vi "20191023_KEK_HEX5_simple.vi"() -> ()   [LabVIEW 2017]
uses:
  <vilib>/DAQmx/create/channels.llb/DAQmx Create Channel (AI-Voltage-Basic).vi
  <vilib>/DAQmx/create/channels.llb/DAQmx Create Channel (AO-Voltage-Basic).vi
  <vilib>/DAQmx/miscellaneous.llb/DAQmx Fill In Error Info.vi
  Lake Shore Cryotronics 218.lvlib
panel:
  out "ref RAW":refnum<file>
  out "ref LSI-D":refnum<file>
  out "ref DAQ":refnum<file>
  in  "CSV filename suffix":string="transfer"
  in  "base path":path=path "C:/Users/TUCAN_rcnp/Desktop/Labview/KEK_20191023_HEX5/EXP"
  out "ref LSI-U":refnum<file>
  out "Cycle #":i32=4
  out "current time":timestamp=timestamp(3655347463.253907 s since 1904-01-01)
  in  "stop":bool
  in  "Tab Control":T1(tab)=enum."config"
  out "error out \n(LSIU)":errorcluster
  out "error out\n(file creation)":errorcluster
  out "error out\n(DAQ config)":errorcluster
  out "error out\n(DAQ OUT)":errorcluster
  out "error out \n(DAQ IN)":errorcluster
  out "error out \n(record LSIU)":errorcluster
  out "error out \n(record DAQ)":errorcluster
  out "error out DAQ close":errorcluster
  out "error out \n(LSID)":errorcluster
  out "error out \n(record LSID)":errorcluster
  out "errors plot cosmetic 1":errorcluster[](array[cluster])
  out "error plot content":errorcluster
  out "error plot cosmetic 2":errorcluster
  in  "comments DAQ (not recorded)":string[](array[string])=["", "", "pressure diff., range : 0-20kPa", "pressure diff., rrange : 0-1kPa", "", "", "The range of this is 0-10VDC", "absoulte pressure, 1-5V <-> 0-200kPa", "absoulte pressure, 1-5V <-> 0-200kPa", "baratron analog out ", "baratron buffer out CDG1", "baratron buffer out CDG1"]
  in  "comments LSID (not recorded)":string[](array[string])=["PtCo", "PtCo", "PtCo", "PtCo", "CERNOX", "CERNOX", "CERNOX", "CERNOX"]
  in  "comments LSIU (not recorded)":string[](array[string])=["PtCo", "", "", "", "CERNOX", "CERNOX", "CERNOX", "CERNOX"]
  in  "V_max(in)":dbl[](array[numeric])=[5.0, 0.15, 5.0, 5.0, 5.0, 5.0, 10.0, 5.0, 5.0, 5.0, 5.0, 5.0]
  in  "NI DAQ AIN labels":string[](array[string])=["P_4KRES", "LM_110", "DP_3He", "DP_4He", "FM_4He", "FM_3He", "LM_1700", "P_3He_IN", "P_3He_OUT", "P_bar_front", "P_bar_CDG1", "P_bar_CDG2"]
  in  "LSI-U CH labels":string[](array[string])=["HEX5_mid", "NC", "NC", "NC", "HEX5_gas_IN", "HEX5_gas_OUT", "JT_IN", "JT_OUT"]
  in  "LSI-D CH labels":string[](array[string])=["Hflex_low", "uper_duct", "Hflex_up", "4K_res_up", "4K_res(broken)", "HEX5_liq_IN", "HEX5_liq_OUT", "1K_pot"]
  in  "DAQ analog channels":tag[](array[tag])=["Dev1/ai1", "Dev1/ai2", "Dev1/ai3", "Dev1/ai4", "Dev1/ai5", "Dev1/ai6", "Dev1/ai7", "Dev1/ai16", "Dev1/ai17", "Dev1/ai18", "Dev1/ai19", "Dev1/ai20"]
  in  "V_min(in)":dbl[](array[numeric])=[0.0, 0.0, 0.0, 0.0, 0.0, 0.0, 0.0, 0.0, 0.0, 0.0, 0.0, 0.0]
  out "DAQ CH OUT":string="O1"
  in  "DAQ  OUT":tag="Dev1/ao0"
  in  "DAQ OUT ON?":bool
  in  "V_min(out)":dbl
  in  "V_max(out)":dbl=5.0
  out "DAQ CH 2":string[](array[string])=["Q1", "Q2", "Q3", "Q4", "Q5", "Q6", "Q7", "Q8", "Q9", "Q10", "Q11", "Q12"]
  out "LSI-D CH 2":string[](array[string])=["D1", "D2", "D3", "D4", "D5", "D6", "D7", "D8"]
  in  "DAQ sample #":i32=5
  out "LSI-U CH 2":string[](array[string])=["U1", "U2", "U3", "U4", "U5", "U6", "U7", "U8"]
  in  "VISA LSI218 UP":refnum<visa-resource-name>="GPIB0::3::INSTR"
  in  "VISA LSI218 DOWN":refnum<visa-resource-name>="GPIB0::11::INSTR"
  out "LSI-D CH indic.":string[](array[string])=["Hflex_low", "uper_duct", "Hflex_up", "4K_res_up", "4K_res(broken)", "HEX5_liq_IN", "HEX5_liq_OUT", "1K_pot"]
  out "LSI-D out":dbl[](array[numeric])=[279.07, 94.738, 115.48, 9.053, 4.259, 7.074, 275.73, 267.7]
  out "D idx":i32[](array[numeric])=[0, 1, 2, 3, 4, 5, 6, 7]
  out "U idx":i32[](array[numeric])=[0, 1, 2, 3, 4, 5, 6, 7]
  out "LSI-U CH indic,":string[](array[string])=["HEX5_mid", "NC", "NC", "NC", "HEX5_gas_IN", "HEX5_gas_OUT", "JT_IN", "JT_OUT"]
  out "LSI-U out":dbl[](array[numeric])=[230.46, 0.0, 330.07, 0.718, 269.26, 40.177, 262.93, 258.86]
  out "Q idx":i32[](array[numeric])=[0, 1, 2, 3, 4, 5, 6, 7, 8, 9, 10, 11]
  out "NI-DAQ CH indic.":string[](array[string])=["P_4KRES", "LM_110", "DP_3He", "DP_4He", "FM_4He", "FM_3He", "LM_1700", "NC", "Bar_anal", "bar_front", "bar_CDG1", "bar_CDG2"]
  out "DAQ CONV. OUT":dbl[](array[numeric])=[102559.43545152312, 99.57724592287158, 8432.483558631859, 1038.356900041269, 58.744507090852395, 0.10776743839642333, 0.25258903935505905, 6023.863022642484, 1254.7840891727778, 1087.5562183651225, 19.65036741849554, 108988.17391753798] format="%#_9f"
  out "RAW (V)":dbl[](array[numeric])=[3.0490844639686365, 0.09946673611804849, 2.685280194879057, 5.153164569644455, 0.5910617469349461, 0.009269963504127919, 0.0080925607634761, 1.124850148957886, 1.0296658437756174, 2.9405843257487403, 0.08735731905919117, 5.447101175410158] format="%#_3f"
  out "DAQ OUT \nsample #":u32=1
  in  "DAQ OUT SET Volt":dbl[](array[numeric])=[2.0] format="%0.2f"
  out "V10 - V8":dbl=2.491326830087994 format="%#_9g"
  out "V9 - V8":dbl=-2.8715405203925584 format="%#_9g"
  out "V10 - V9":dbl=5.362867350480552 format="%#_9g"
  in  "Bar_anal Vbar offset":dbl format="%#_7g"
  in  "Bar_CDG1 Vbar offset":dbl=-2.0 format="%#_7g"
  in  "Bar_CDG2 Vbar offset":dbl=1.490863 format="%#_7g"
  out "Graph LSI-D 1":cluster{dbl[], dbl[]}[](graph)=[{[3655347443.2539887, 3655347448.2538176, 3655347453.25365, 3655347458.2533135, 3655347463.253907], [0.0, 279.03, 279.08, 279.06, 279.07]}, {[3655347443.2539887, 3655347448.2538176, 3655347453.25365, 3655347458.2533135, 3655347463.253907], [0.0, 94.941, 94.88, 94.814, 94.738]}, {[3655347443.2539887, 3655347448.2538176, 3655347453.25365, 3655347458.2533135, 3655347463.253907], [0.0, 115.54, 115.51, 115.5, 115.48]}, {[3655347443.2539887, 3655347448.2538176, 3655347453.25365, 3655347458.2533135, 3655347463.253907], [0.0, 9.048, 9.057, 9.053, 9.053]}, {[3655347443.2539887, 3655347448.2538176, 3655347453.25365, 3655347458.2533135, 3655347463.253907], [0.0, 4.26, 4.26, 4.26, 4.259]}, {[3655347443.2539887, 3655347448.2538176, 3655347453.25365, 3655347458.2533135, 3655347463.253907], [0.0, 7.078, 7.076, 7.076, 7.074]}, {[3655347443.2539887, 3655347448.2538176, 3655347453.25365, 3655347458.2533135, 3655347463.253907], [0.0, 275.75, 275.79, 275.79, 275.73]}, {[3655347443.2539887, 3655347448.2538176, 3655347453.25365, 3655347458.2533135, 3655347463.253907], [0.0, 268.38, 269.57, 269.92, 267.7]}, {[3655347443.2539887, 3655347448.2538176, 3655347453.25365, 3655347458.2533135, 3655347463.253907], []}] caption="XY Graph"
  out "LSI-U out 1":dbl[](array[numeric])=[230.46, 0.0, 330.07, 0.718, 269.26, 40.177, 262.93, 258.86] format="%_3f"
  out "Graph LSI-U 1":cluster{dbl[], dbl[]}[](graph)=[{[3655347443.2539887, 3655347448.2538176, 3655347453.25365, 3655347458.2533135, 3655347463.253907], [230.43, 230.43, 230.46, 230.44, 230.46]}, {[3655347443.2539887, 3655347448.2538176, 3655347453.25365, 3655347458.2533135, 3655347463.253907], [0.0, 0.0, 0.0, 0.0, 0.0]}, {[3655347443.2539887, 3655347448.2538176, 3655347453.25365, 3655347458.2533135, 3655347463.253907], [330.07, 330.07, 330.07, 330.07, 330.07]}, {[3655347443.2539887, 3655347448.2538176, 3655347453.25365, 3655347458.2533135, 3655347463.253907], [0.718, 0.718, 0.718, 0.718, 0.718]}, {[3655347443.2539887, 3655347448.2538176, 3655347453.25365, 3655347458.2533135, 3655347463.253907], [269.04, 268.77, 267.57, 267.77, 269.26]}, {[3655347443.2539887, 3655347448.2538176, 3655347453.25365, 3655347458.2533135, 3655347463.253907], [41.126, 41.053, 40.912, 40.409, 40.177]}, {[3655347443.2539887, 3655347448.2538176, 3655347453.25365, 3655347458.2533135, 3655347463.253907], [263.91, 263.46, 264.61, 264.6, 262.93]}, {[3655347443.2539887, 3655347448.2538176, 3655347453.25365, 3655347458.2533135, 3655347463.253907], [258.41, 256.34, 256.5, 259.99, 258.86]}, {[3655347443.2539887, 3655347448.2538176, 3655347453.25365, 3655347458.2533135, 3655347463.253907], []}] caption="XY Graph"
  out "Graph LSI-U 2":cluster{dbl[], dbl[]}[](graph)=[{[3655347443.2539887, 3655347448.2538176, 3655347453.25365, 3655347458.2533135, 3655347463.253907], [230.43, 230.43, 230.46, 230.44, 230.46]}, {[3655347443.2539887, 3655347448.2538176, 3655347453.25365, 3655347458.2533135, 3655347463.253907], [0.0, 0.0, 0.0, 0.0, 0.0]}, {[3655347443.2539887, 3655347448.2538176, 3655347453.25365, 3655347458.2533135, 3655347463.253907], [330.07, 330.07, 330.07, 330.07, 330.07]}, {[3655347443.2539887, 3655347448.2538176, 3655347453.25365, 3655347458.2533135, 3655347463.253907], [0.718, 0.718, 0.718, 0.718, 0.718]}, {[3655347443.2539887, 3655347448.2538176, 3655347453.25365, 3655347458.2533135, 3655347463.253907], [269.04, 268.77, 267.57, 267.77, 269.26]}, {[3655347443.2539887, 3655347448.2538176, 3655347453.25365, 3655347458.2533135, 3655347463.253907], [41.126, 41.053, 40.912, 40.409, 40.177]}, {[3655347443.2539887, 3655347448.2538176, 3655347453.25365, 3655347458.2533135, 3655347463.253907], [263.91, 263.46, 264.61, 264.6, 262.93]}, {[3655347443.2539887, 3655347448.2538176, 3655347453.25365, 3655347458.2533135, 3655347463.253907], [258.41, 256.34, 256.5, 259.99, 258.86]}, {[3655347443.2539887, 3655347448.2538176, 3655347453.25365, 3655347458.2533135, 3655347463.253907], []}] caption="XY Graph"
  out "LSI-U out 2":dbl[](array[numeric])=[230.46, 0.0, 330.07, 0.718, 269.26, 40.177, 262.93, 258.86] format="%_3f"
  out "Graph LSI-D 2":cluster{dbl[], dbl[]}[](graph)=[{[3655347443.2539887, 3655347448.2538176, 3655347453.25365, 3655347458.2533135, 3655347463.253907], [0.0, 279.03, 279.08, 279.06, 279.07]}, {[3655347443.2539887, 3655347448.2538176, 3655347453.25365, 3655347458.2533135, 3655347463.253907], [0.0, 94.941, 94.88, 94.814, 94.738]}, {[3655347443.2539887, 3655347448.2538176, 3655347453.25365, 3655347458.2533135, 3655347463.253907], [0.0, 115.54, 115.51, 115.5, 115.48]}, {[3655347443.2539887, 3655347448.2538176, 3655347453.25365, 3655347458.2533135, 3655347463.253907], [0.0, 9.048, 9.057, 9.053, 9.053]}, {[3655347443.2539887, 3655347448.2538176, 3655347453.25365, 3655347458.2533135, 3655347463.253907], [0.0, 4.26, 4.26, 4.26, 4.259]}, {[3655347443.2539887, 3655347448.2538176, 3655347453.25365, 3655347458.2533135, 3655347463.253907], [0.0, 7.078, 7.076, 7.076, 7.074]}, {[3655347443.2539887, 3655347448.2538176, 3655347453.25365, 3655347458.2533135, 3655347463.253907], [0.0, 275.75, 275.79, 275.79, 275.73]}, {[3655347443.2539887, 3655347448.2538176, 3655347453.25365, 3655347458.2533135, 3655347463.253907], [0.0, 268.38, 269.57, 269.92, 267.7]}, {[3655347443.2539887, 3655347448.2538176, 3655347453.25365, 3655347458.2533135, 3655347463.253907], []}] caption="XY Graph"
  out "LSI-D out 2":dbl[](array[numeric])=[279.07, 94.738, 115.48, 9.053, 4.259, 7.074, 275.73, 267.7] format="%_3f"
  out "LSI-D out 1":dbl[](array[numeric])=[279.07, 94.738, 115.48, 9.053, 4.259, 7.074, 275.73, 267.7] format="%_3f"
  out "OUT S.4":dbl[](array[numeric])=[102559.43545152312, 99.57724592287158, 8432.483558631859, 1038.356900041269, 58.744507090852395, 0.10776743839642333, 0.25258903935505905, 6023.863022642484, 1254.7840891727778, 1087.5562183651225, 19.65036741849554, 108988.17391753798] format="%_4e"
  out "XY Graph S.4":cluster{dbl[], dbl[]}[](graph)=[{[3655347443.2539887, 3655347448.2538176, 3655347453.25365, 3655347458.2533135, 3655347463.253907], [102690.95076766326, 102848.76914703452, 102467.37472998732, 102608.75369506289, 102559.43545152312]}, {[3655347443.2539887, 3655347448.2538176, 3655347453.25365, 3655347458.2533135, 3655347463.253907], [99.39569409811979, 99.95350549692311, 99.32859886094775, 99.43647748010623, 99.57724592287158]}, {[3655347443.2539887, 3655347448.2538176, 3655347453.25365, 3655347458.2533135, 3655347463.253907], [8424.921426873496, 8447.44342794192, 8435.607047832149, 8442.347208739231, 8432.483558631859]}, {[3655347443.2539887, 3655347448.2538176, 3655347453.25365, 3655347458.2533135, 3655347463.253907], [1037.0992853630753, 1038.6528093772615, 1037.6171267012242, 1038.324021226166, 1038.356900041269]}, {[3655347443.2539887, 3655347448.2538176, 3655347453.25365, 3655347458.2533135, 3655347463.253907], [59.060144270787106, 58.829992160378474, 58.45517300795377, 58.75108286532355, 58.744507090852395]}, {[3655347443.2539887, 3655347448.2538176, 3655347453.25365, 3655347458.2533135, 3655347463.253907], [0.022282330072040446, 0.07357339545420755, 0.1564281925601952, 0.08277948378294703, 0.10776743839642333]}, {[3655347443.2539887, 3655347448.2538176, 3655347453.25365, 3655347458.2533135, 3655347463.253907], [6101.12834589025, 6130.719320780331, 6140.582979028531, 5979.4765600999945, 6023.863022642484]}, {[3655347443.2539887, 3655347448.2538176, 3655347453.25365, 3655347458.2533135, 3655347463.253907], [0.08750275072771002, 0.08618732210876909, 0.08355646487079943, 0.07632160746464861, 0.25258903935505905]}, {[3655347443.2539887, 3655347448.2538176, 3655347453.25365, 3655347458.2533135, 3655347463.253907], [1156.1474997572097, 958.8743208872041, 940.7909480054877, 819.1391531159998, 1254.7840891727778]}, {[3655347443.2539887, 3655347448.2538176, 3655347453.25365, 3655347458.2533135, 3655347463.253907], [1088.0503397791224, 1107.1618683137349, 1103.479962198376, 1084.7604328484829, 1087.5562183651225]}, {[3655347443.2539887, 3655347448.2538176, 3655347453.25365, 3655347458.2533135, 3655347463.253907], [19.78171848354259, 19.754779982466093, 19.452028824997335, 19.393212177890806, 19.65036741849554]}, {[3655347443.2539887, 3655347448.2538176, 3655347453.25365, 3655347458.2533135, 3655347463.253907], [108988.17391753798, 108988.17391753798, 108988.17391753798, 108988.17391753798, 108988.17391753798]}] caption="XY Graph"
  in  "log/linear 4":bool=TRUE
  out "XY Graph S.3":cluster{dbl[], dbl[]}[](graph)=[{[3655347443.2539887, 3655347448.2538176, 3655347453.25365, 3655347458.2533135, 3655347463.253907], [102690.95076766326, 102848.76914703452, 102467.37472998732, 102608.75369506289, 102559.43545152312]}, {[3655347443.2539887, 3655347448.2538176, 3655347453.25365, 3655347458.2533135, 3655347463.253907], [99.39569409811979, 99.95350549692311, 99.32859886094775, 99.43647748010623, 99.57724592287158]}, {[3655347443.2539887, 3655347448.2538176, 3655347453.25365, 3655347458.2533135, 3655347463.253907], [8424.921426873496, 8447.44342794192, 8435.607047832149, 8442.347208739231, 8432.483558631859]}, {[3655347443.2539887, 3655347448.2538176, 3655347453.25365, 3655347458.2533135, 3655347463.253907], [1037.0992853630753, 1038.6528093772615, 1037.6171267012242, 1038.324021226166, 1038.356900041269]}, {[3655347443.2539887, 3655347448.2538176, 3655347453.25365, 3655347458.2533135, 3655347463.253907], [59.060144270787106, 58.829992160378474, 58.45517300795377, 58.75108286532355, 58.744507090852395]}, {[3655347443.2539887, 3655347448.2538176, 3655347453.25365, 3655347458.2533135, 3655347463.253907], [0.022282330072040446, 0.07357339545420755, 0.1564281925601952, 0.08277948378294703, 0.10776743839642333]}, {[3655347443.2539887, 3655347448.2538176, 3655347453.25365, 3655347458.2533135, 3655347463.253907], [6101.12834589025, 6130.719320780331, 6140.582979028531, 5979.4765600999945, 6023.863022642484]}, {[3655347443.2539887, 3655347448.2538176, 3655347453.25365, 3655347458.2533135, 3655347463.253907], [0.08750275072771002, 0.08618732210876909, 0.08355646487079943, 0.07632160746464861, 0.25258903935505905]}, {[3655347443.2539887, 3655347448.2538176, 3655347453.25365, 3655347458.2533135, 3655347463.253907], [1156.1474997572097, 958.8743208872041, 940.7909480054877, 819.1391531159998, 1254.7840891727778]}, {[3655347443.2539887, 3655347448.2538176, 3655347453.25365, 3655347458.2533135, 3655347463.253907], [1088.0503397791224, 1107.1618683137349, 1103.479962198376, 1084.7604328484829, 1087.5562183651225]}, {[3655347443.2539887, 3655347448.2538176, 3655347453.25365, 3655347458.2533135, 3655347463.253907], [19.78171848354259, 19.754779982466093, 19.452028824997335, 19.393212177890806, 19.65036741849554]}, {[3655347443.2539887, 3655347448.2538176, 3655347453.25365, 3655347458.2533135, 3655347463.253907], [108988.17391753798, 108988.17391753798, 108988.17391753798, 108988.17391753798, 108988.17391753798]}] caption="XY Graph"
  in  "log/linear 3":bool=TRUE
  out "XY Graph S.2":cluster{dbl[], dbl[]}[](graph)=[{[3655347443.2539887, 3655347448.2538176, 3655347453.25365, 3655347458.2533135, 3655347463.253907], [102690.95076766326, 102848.76914703452, 102467.37472998732, 102608.75369506289, 102559.43545152312]}, {[3655347443.2539887, 3655347448.2538176, 3655347453.25365, 3655347458.2533135, 3655347463.253907], [99.39569409811979, 99.95350549692311, 99.32859886094775, 99.43647748010623, 99.57724592287158]}, {[3655347443.2539887, 3655347448.2538176, 3655347453.25365, 3655347458.2533135, 3655347463.253907], [8424.921426873496, 8447.44342794192, 8435.607047832149, 8442.347208739231, 8432.483558631859]}, {[3655347443.2539887, 3655347448.2538176, 3655347453.25365, 3655347458.2533135, 3655347463.253907], [1037.0992853630753, 1038.6528093772615, 1037.6171267012242, 1038.324021226166, 1038.356900041269]}, {[3655347443.2539887, 3655347448.2538176, 3655347453.25365, 3655347458.2533135, 3655347463.253907], [59.060144270787106, 58.829992160378474, 58.45517300795377, 58.75108286532355, 58.744507090852395]}, {[3655347443.2539887, 3655347448.2538176, 3655347453.25365, 3655347458.2533135, 3655347463.253907], [0.022282330072040446, 0.07357339545420755, 0.1564281925601952, 0.08277948378294703, 0.10776743839642333]}, {[3655347443.2539887, 3655347448.2538176, 3655347453.25365, 3655347458.2533135, 3655347463.253907], [6101.12834589025, 6130.719320780331, 6140.582979028531, 5979.4765600999945, 6023.863022642484]}, {[3655347443.2539887, 3655347448.2538176, 3655347453.25365, 3655347458.2533135, 3655347463.253907], [0.08750275072771002, 0.08618732210876909, 0.08355646487079943, 0.07632160746464861, 0.25258903935505905]}, {[3655347443.2539887, 3655347448.2538176, 3655347453.25365, 3655347458.2533135, 3655347463.253907], [1156.1474997572097, 958.8743208872041, 940.7909480054877, 819.1391531159998, 1254.7840891727778]}, {[3655347443.2539887, 3655347448.2538176, 3655347453.25365, 3655347458.2533135, 3655347463.253907], [1088.0503397791224, 1107.1618683137349, 1103.479962198376, 1084.7604328484829, 1087.5562183651225]}, {[3655347443.2539887, 3655347448.2538176, 3655347453.25365, 3655347458.2533135, 3655347463.253907], [19.78171848354259, 19.754779982466093, 19.452028824997335, 19.393212177890806, 19.65036741849554]}, {[3655347443.2539887, 3655347448.2538176, 3655347453.25365, 3655347458.2533135, 3655347463.253907], [108988.17391753798, 108988.17391753798, 108988.17391753798, 108988.17391753798, 108988.17391753798]}] caption="XY Graph"
  in  "log/linear 2":bool=TRUE
  out "OUT S.2":dbl[](array[numeric])=[102559.43545152312, 99.57724592287158, 8432.483558631859, 1038.356900041269, 58.744507090852395, 0.10776743839642333, 0.25258903935505905, 6023.863022642484, 1254.7840891727778, 1087.5562183651225, 19.65036741849554, 108988.17391753798] format="%_4e"
  in  "log/linear 1":bool=TRUE
  out "OUT S.1":dbl[](array[numeric])=[102559.43545152312, 99.57724592287158, 8432.483558631859, 1038.356900041269, 58.744507090852395, 0.10776743839642333, 0.25258903935505905, 6023.863022642484, 1254.7840891727778, 1087.5562183651225, 19.65036741849554, 108988.17391753798] format="%_4e"
  out "OUT S.3":dbl[](array[numeric])=[102559.43545152312, 99.57724592287158, 8432.483558631859, 1038.356900041269, 58.744507090852395, 0.10776743839642333, 0.25258903935505905, 6023.863022642484, 1254.7840891727778, 1087.5562183651225, 19.65036741849554, 108988.17391753798] format="%_4e"
  out "XY Graph S.1":cluster{dbl[], dbl[]}[](graph)=[{[3655347443.2539887, 3655347448.2538176, 3655347453.25365, 3655347458.2533135, 3655347463.253907], [102690.95076766326, 102848.76914703452, 102467.37472998732, 102608.75369506289, 102559.43545152312]}, {[3655347443.2539887, 3655347448.2538176, 3655347453.25365, 3655347458.2533135, 3655347463.253907], [99.39569409811979, 99.95350549692311, 99.32859886094775, 99.43647748010623, 99.57724592287158]}, {[3655347443.2539887, 3655347448.2538176, 3655347453.25365, 3655347458.2533135, 3655347463.253907], [8424.921426873496, 8447.44342794192, 8435.607047832149, 8442.347208739231, 8432.483558631859]}, {[3655347443.2539887, 3655347448.2538176, 3655347453.25365, 3655347458.2533135, 3655347463.253907], [1037.0992853630753, 1038.6528093772615, 1037.6171267012242, 1038.324021226166, 1038.356900041269]}, {[3655347443.2539887, 3655347448.2538176, 3655347453.25365, 3655347458.2533135, 3655347463.253907], [59.060144270787106, 58.829992160378474, 58.45517300795377, 58.75108286532355, 58.744507090852395]}, {[3655347443.2539887, 3655347448.2538176, 3655347453.25365, 3655347458.2533135, 3655347463.253907], [0.022282330072040446, 0.07357339545420755, 0.1564281925601952, 0.08277948378294703, 0.10776743839642333]}, {[3655347443.2539887, 3655347448.2538176, 3655347453.25365, 3655347458.2533135, 3655347463.253907], [6101.12834589025, 6130.719320780331, 6140.582979028531, 5979.4765600999945, 6023.863022642484]}, {[3655347443.2539887, 3655347448.2538176, 3655347453.25365, 3655347458.2533135, 3655347463.253907], [0.08750275072771002, 0.08618732210876909, 0.08355646487079943, 0.07632160746464861, 0.25258903935505905]}, {[3655347443.2539887, 3655347448.2538176, 3655347453.25365, 3655347458.2533135, 3655347463.253907], [1156.1474997572097, 958.8743208872041, 940.7909480054877, 819.1391531159998, 1254.7840891727778]}, {[3655347443.2539887, 3655347448.2538176, 3655347453.25365, 3655347458.2533135, 3655347463.253907], [1088.0503397791224, 1107.1618683137349, 1103.479962198376, 1084.7604328484829, 1087.5562183651225]}, {[3655347443.2539887, 3655347448.2538176, 3655347453.25365, 3655347458.2533135, 3655347463.253907], [19.78171848354259, 19.754779982466093, 19.452028824997335, 19.393212177890806, 19.65036741849554]}, {[3655347443.2539887, 3655347448.2538176, 3655347453.25365, 3655347458.2533135, 3655347463.253907], [108988.17391753798, 108988.17391753798, 108988.17391753798, 108988.17391753798, 108988.17391753798]}] caption="XY Graph"
  out "date/time string":string="20191031_151722_"
  in  "Wait (s)":i32=5
  # "Record Config"
  # "Some time needed until program stops!"
  # "Error states"
  # "Inputs on this page have to be filled before the start of the program"
  # "LSI VISA addresses"
  # "Defines # of measurements \n taken for averaging\n (only ested with 5!)"
  # "NI DAQ OUT"
  # "LSI-U"
  # "LSI-D"
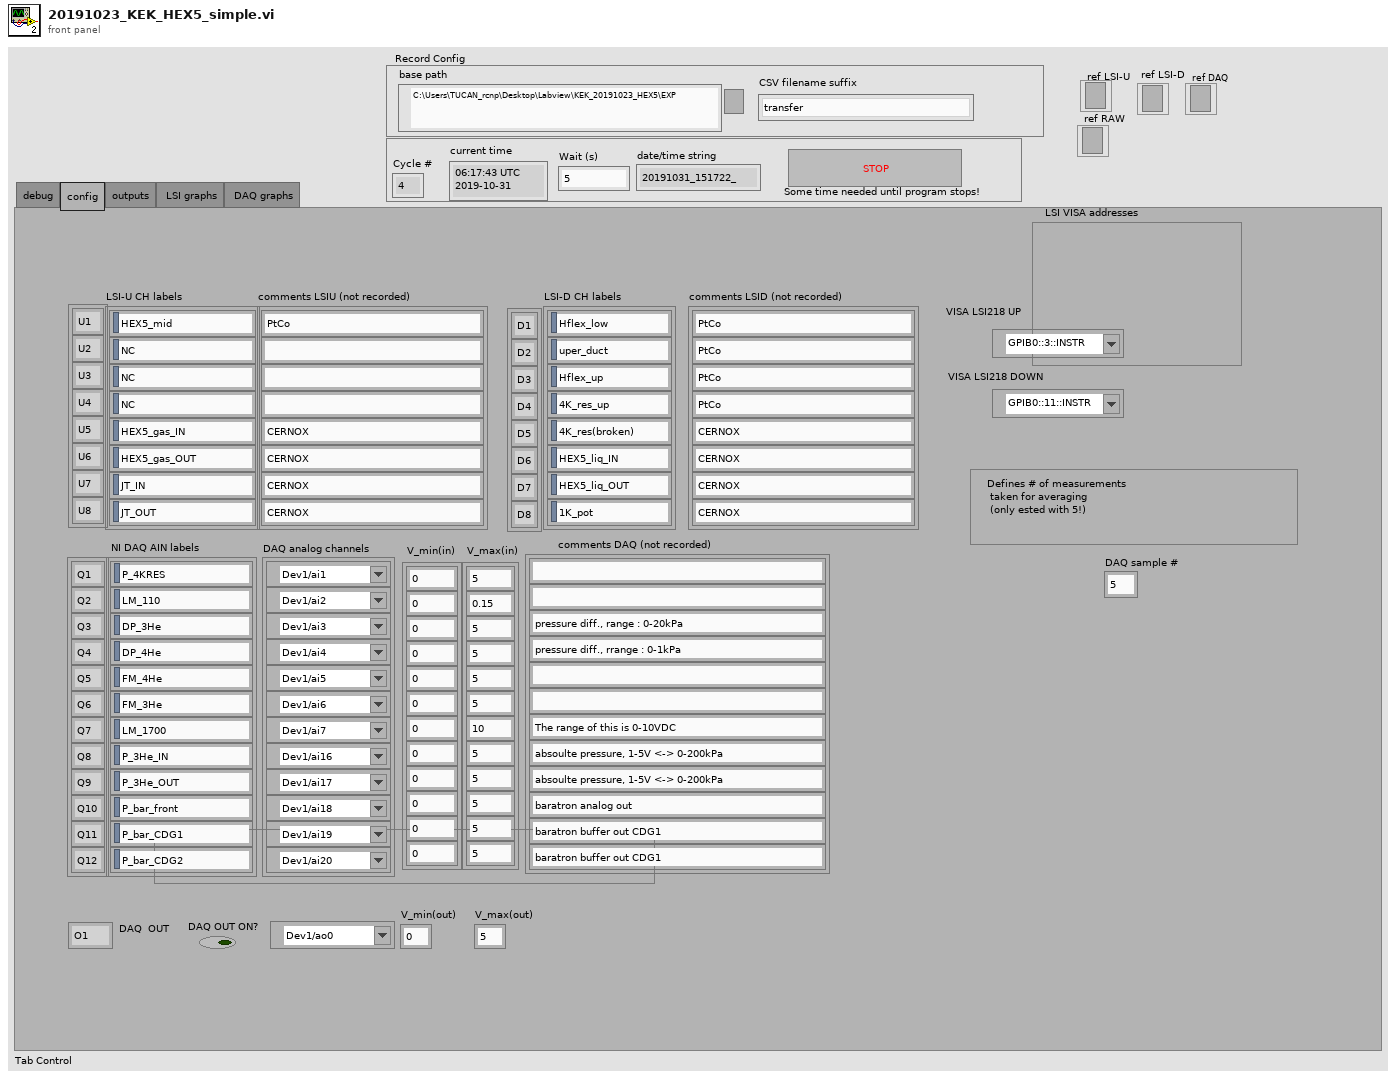
[diagram p1: front panel]
types:
  T1 = enum32{"debug", "config", "outputs", " LSI graphs", " DAQ graphs"}
  T2 = enum16{"open", "replace", "create", "open or create", "replace or create", "replace or create with confirmation"}
  T3 = cluster{"LSI-U CH labels[0]":string, "LSI-U CH labels[1]":string, "LSI-U CH labels[2]":string, "LSI-U CH labels[3]":string, "LSI-U CH labels[4]":string, "LSI-U CH labels[5]":string, "LSI-U CH labels[6]":string, "LSI-U CH labels[7]":string, "LSI-U CH labels[8]":string}
  T4 = cluster{"LSI-D CH labels[0]":string, "LSI-D CH labels[1]":string, "LSI-D CH labels[2]":string, "LSI-D CH labels[3]":string, "LSI-D CH labels[4]":string, "LSI-D CH labels[5]":string, "LSI-D CH labels[6]":string, "LSI-D CH labels[7]":string, "LSI-D CH labels[8]":string}
  T5 = cluster{"LSI-D out[0]":dbl, "LSI-D out[1]":dbl, "LSI-D out[2]":dbl, "LSI-D out[3]":dbl, "LSI-D out[4]":dbl, "LSI-D out[5]":dbl, "LSI-D out[6]":dbl, "LSI-D out[7]":dbl, "LSI-D out[8]":dbl}
  T6 = cluster{"LSI-U out[0]":dbl, "LSI-U out[1]":dbl, "LSI-U out[2]":dbl, "LSI-U out[3]":dbl, "LSI-U out[4]":dbl, "LSI-U out[5]":dbl, "LSI-U out[6]":dbl, "LSI-U out[7]":dbl, "LSI-U out[8]":dbl}
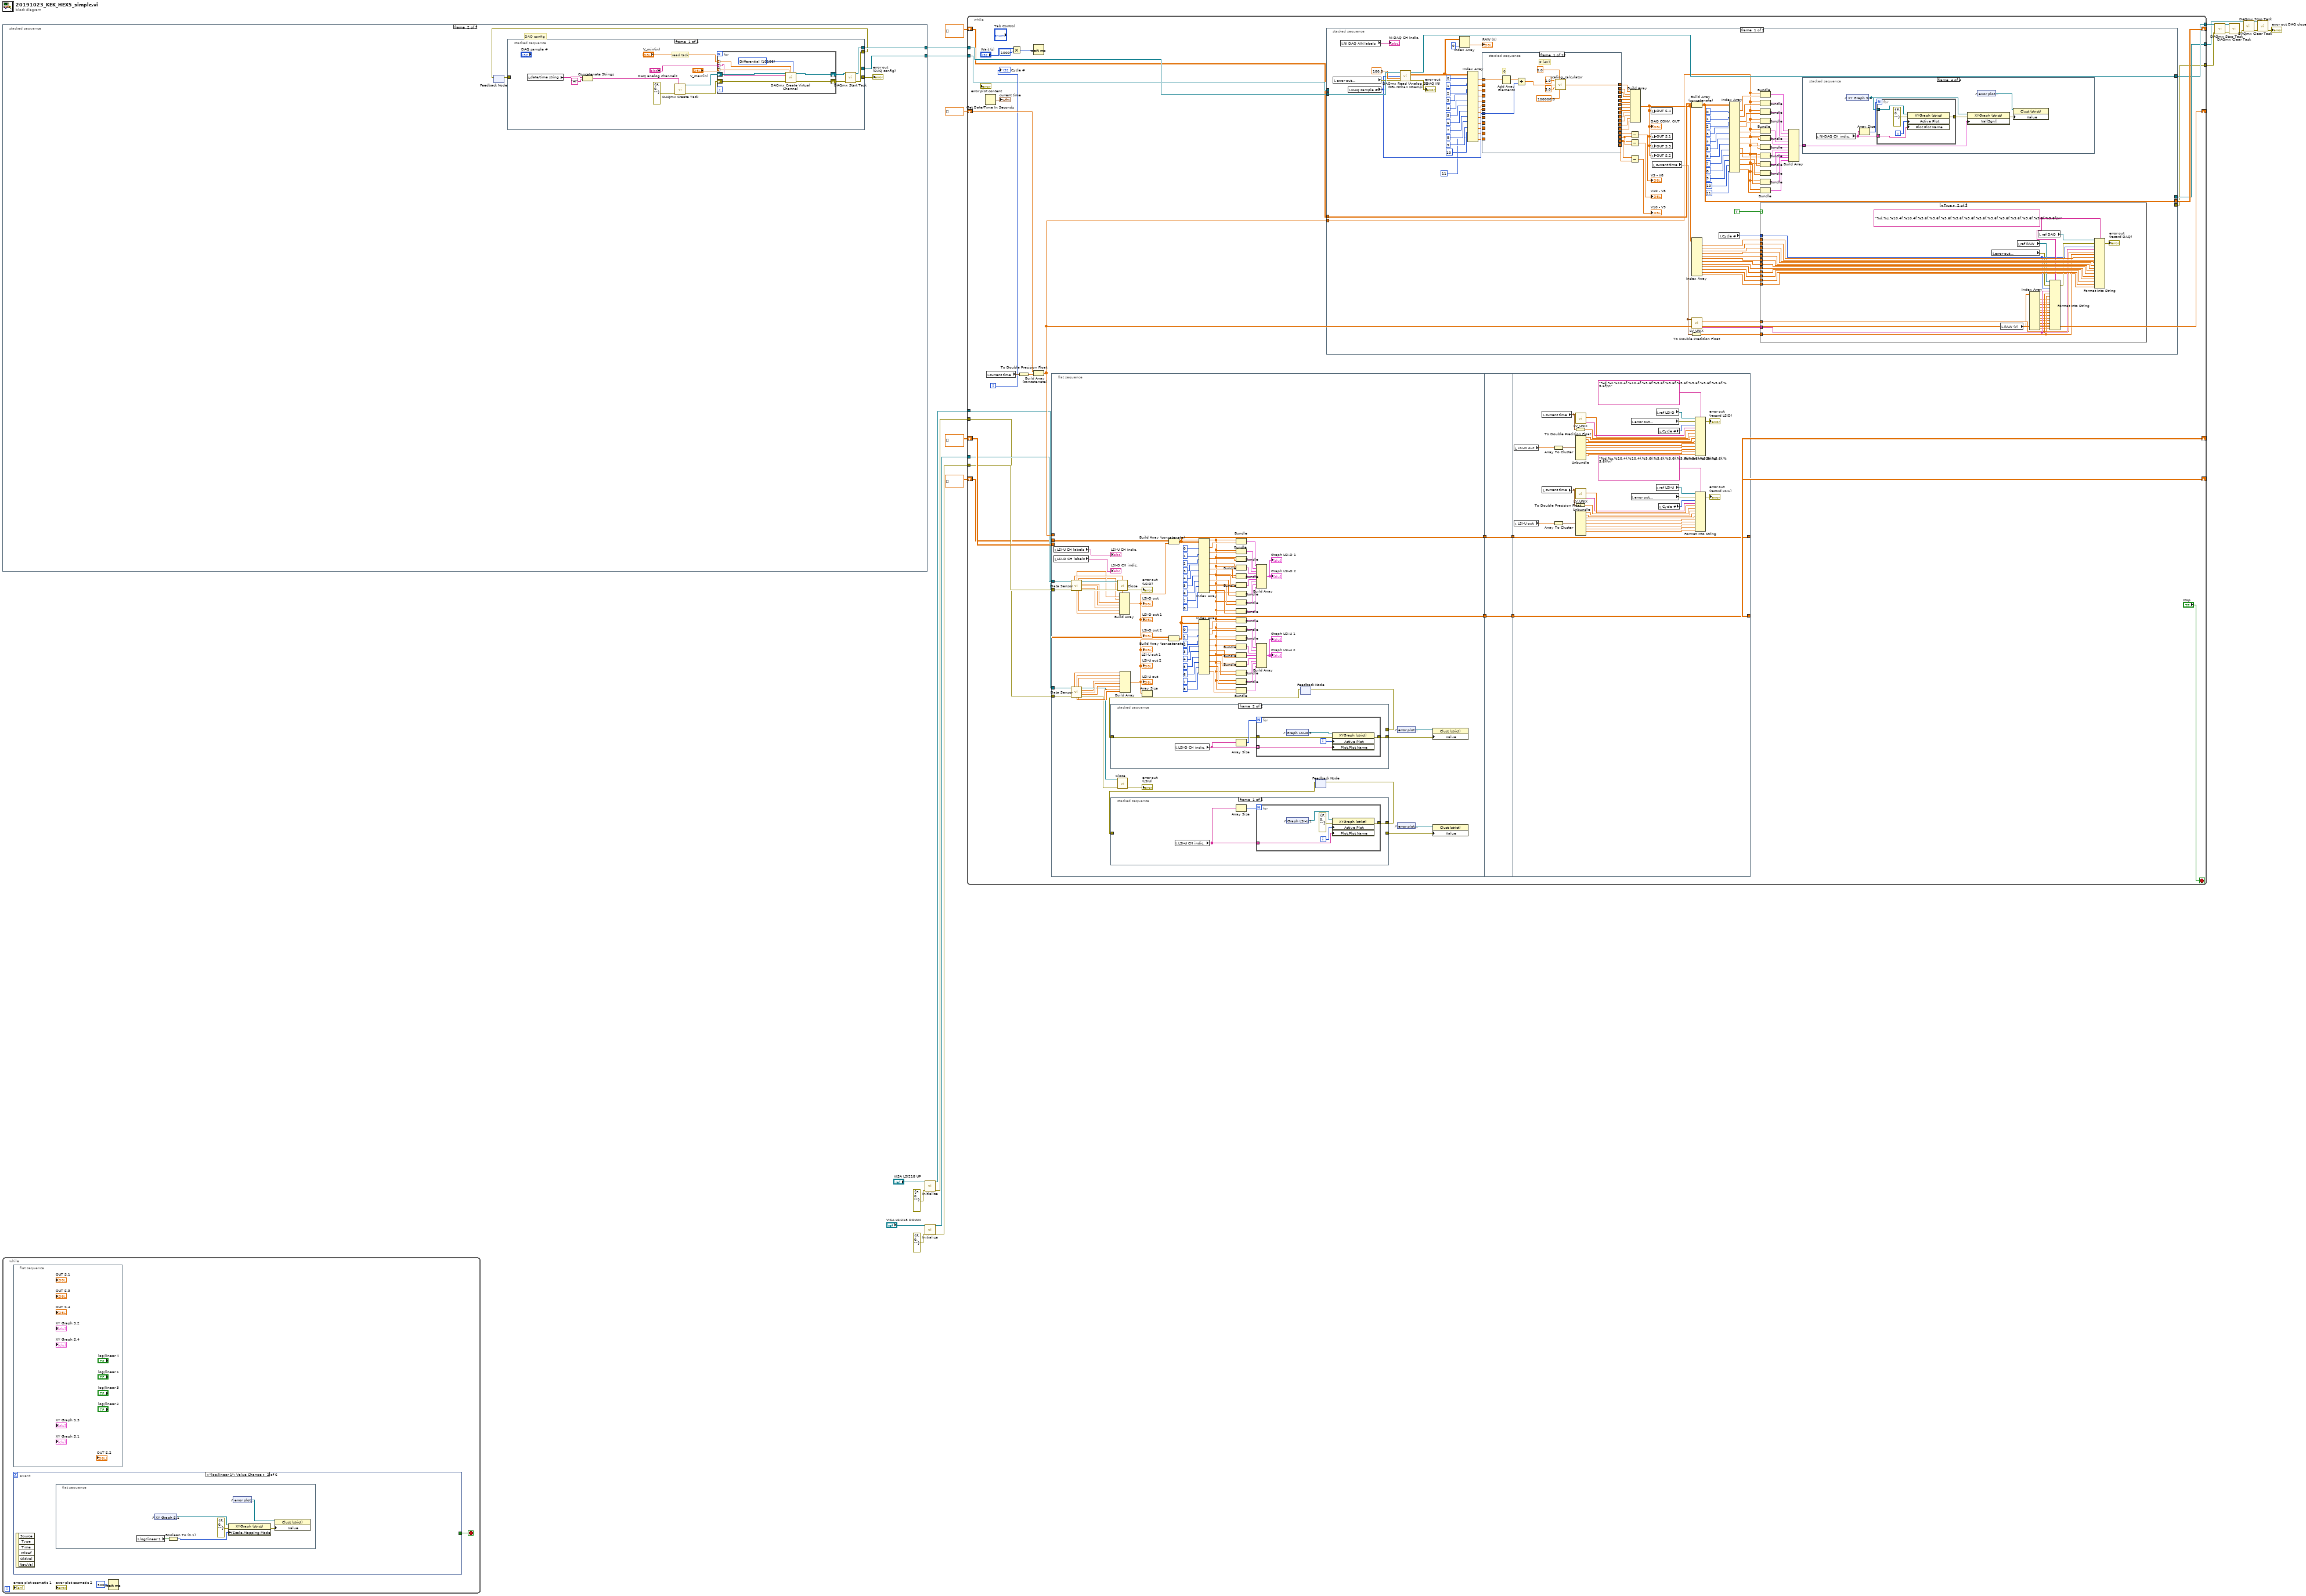
[diagram p0: block diagram]
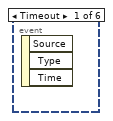
[diagram p2: hidden frame]
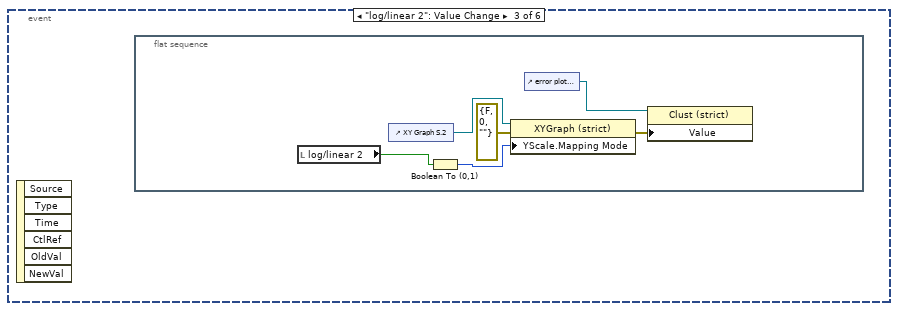
[diagram p3: hidden frame]
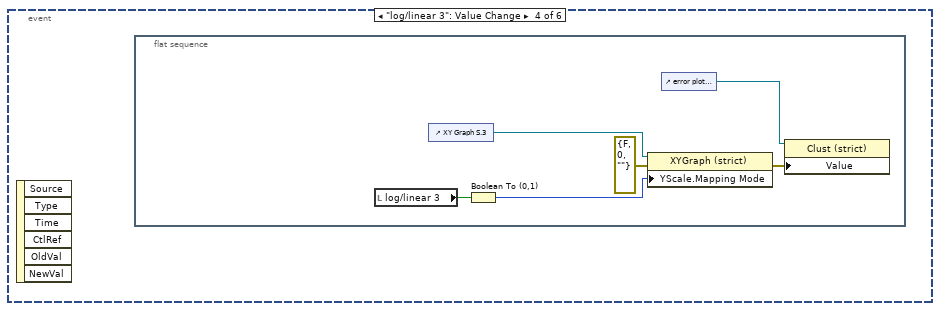
[diagram p4: hidden frame]
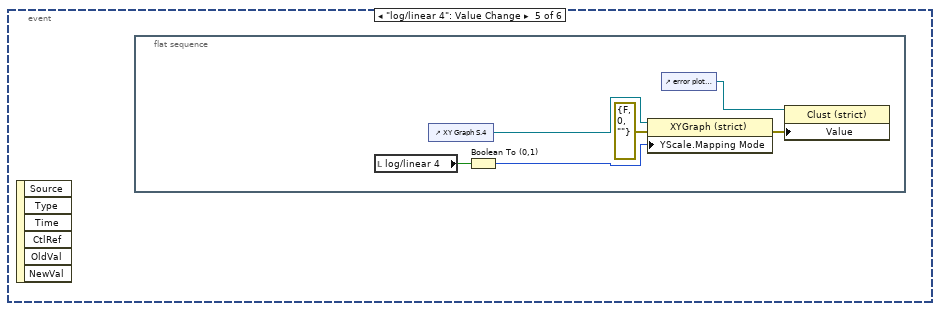
[diagram p5: hidden frame]
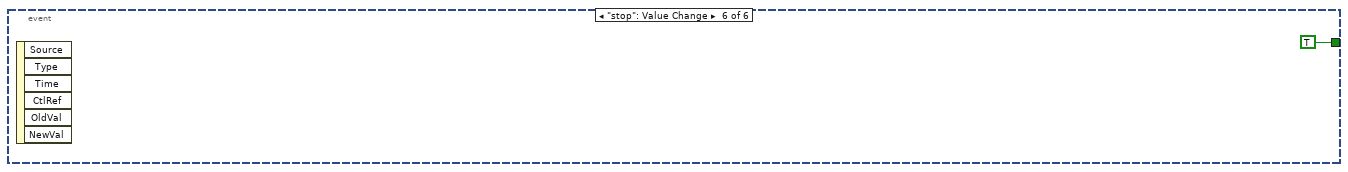
[diagram p6: hidden frame]
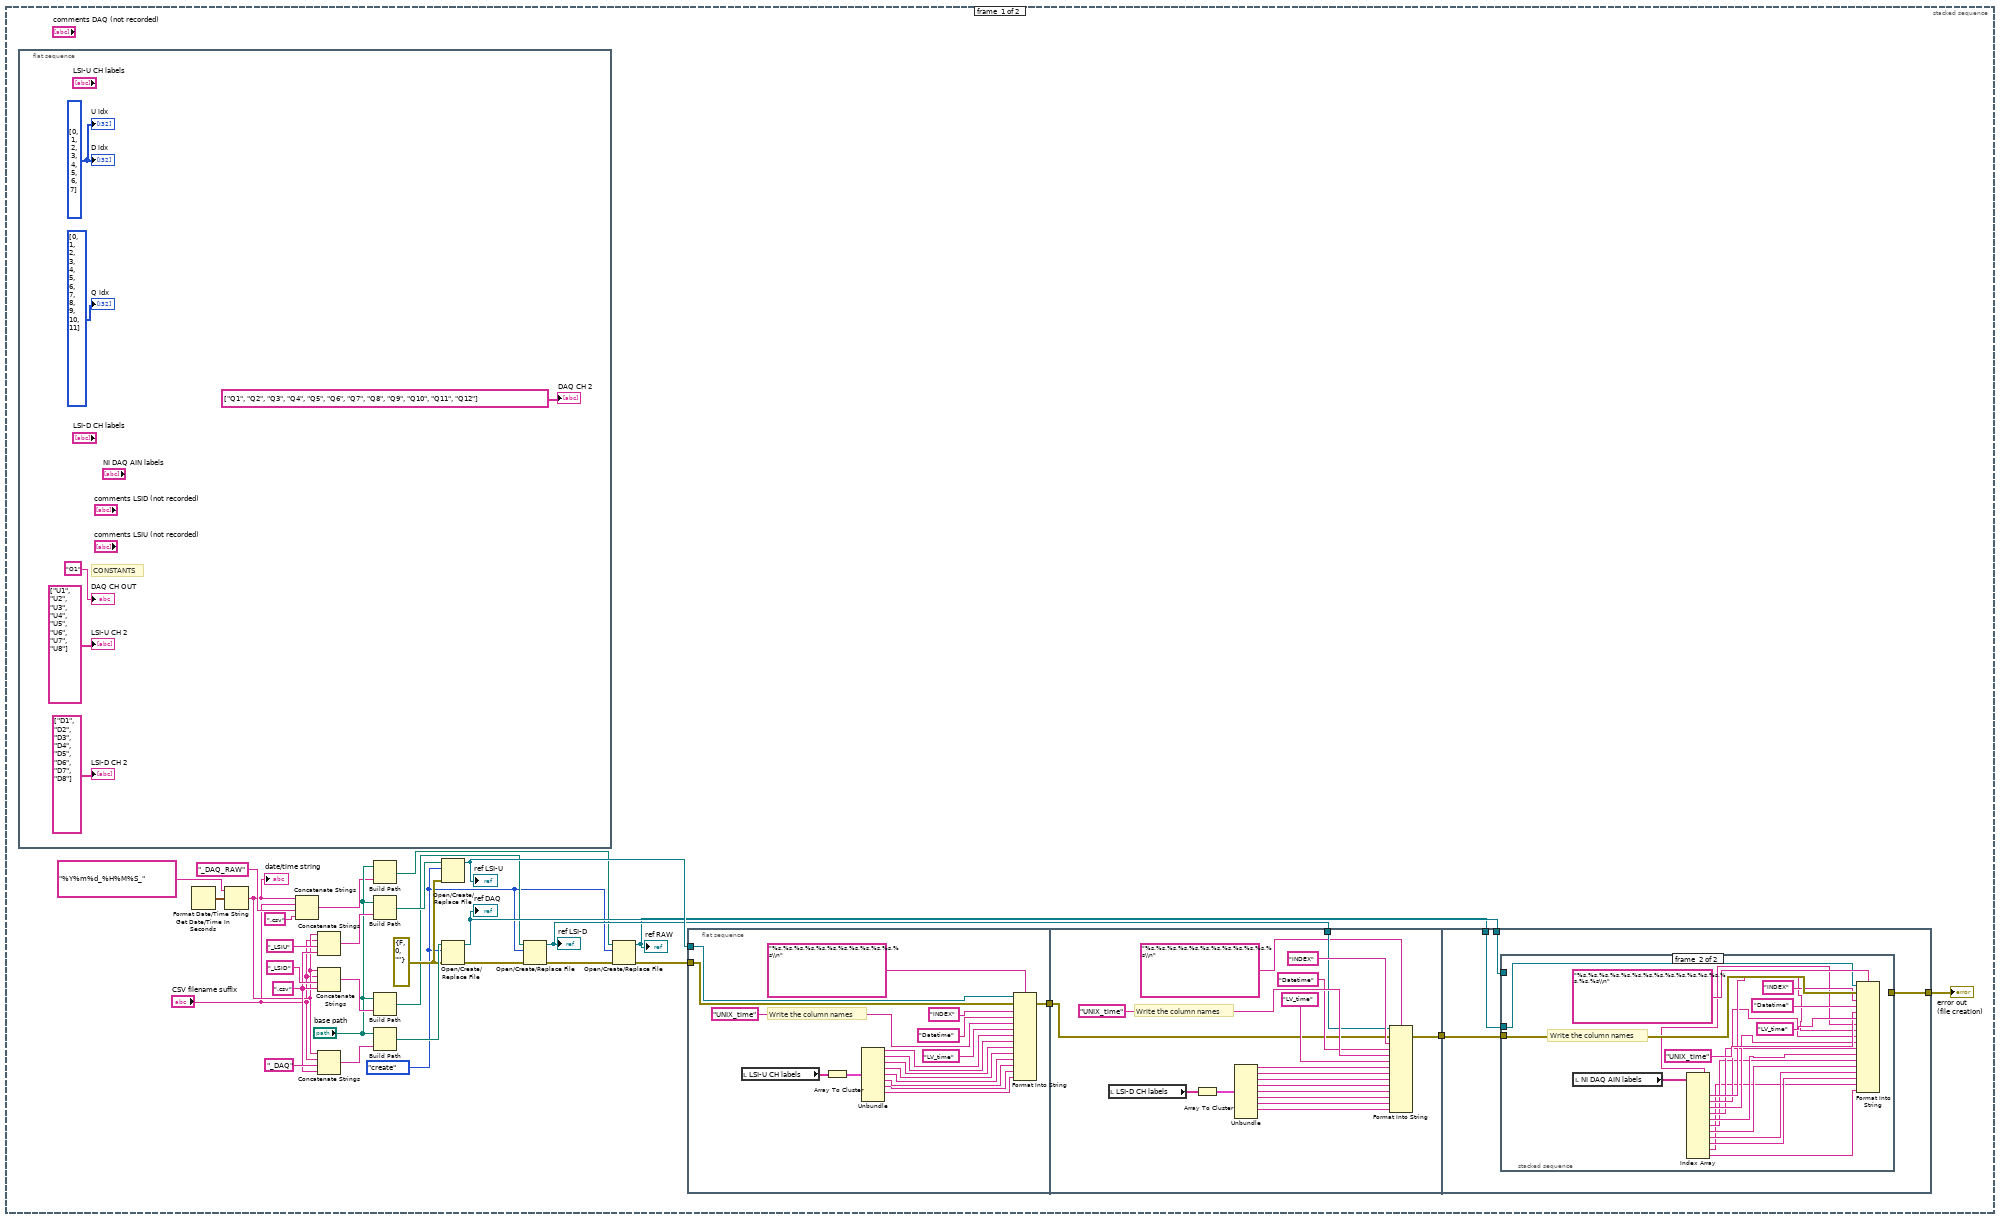
[diagram p7: hidden frame]
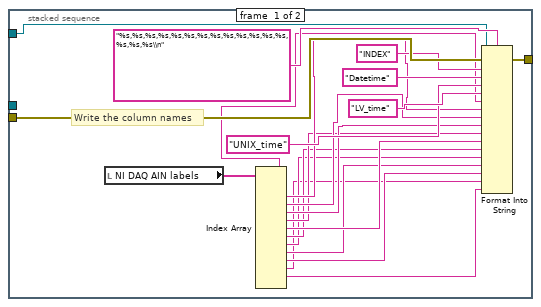
[diagram p8: hidden frame]
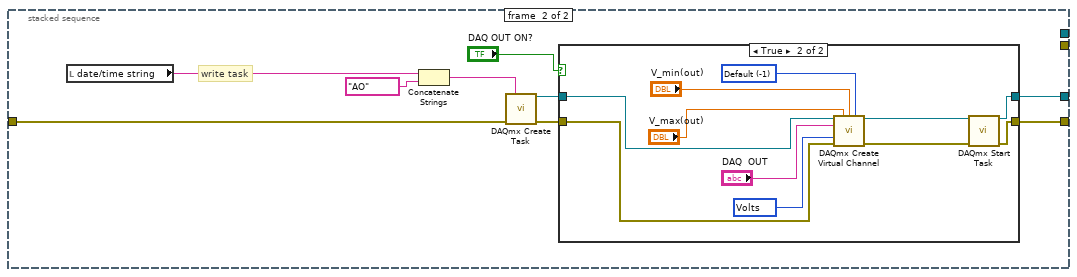
[diagram p9: hidden frame]
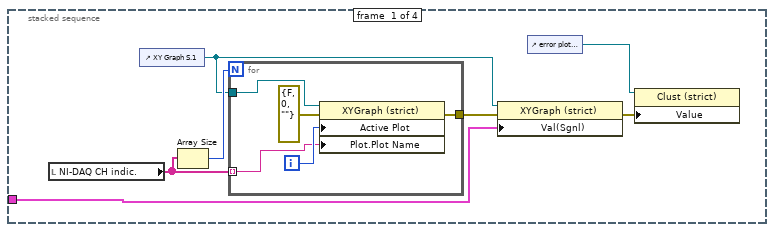
[diagram p12: hidden frame]
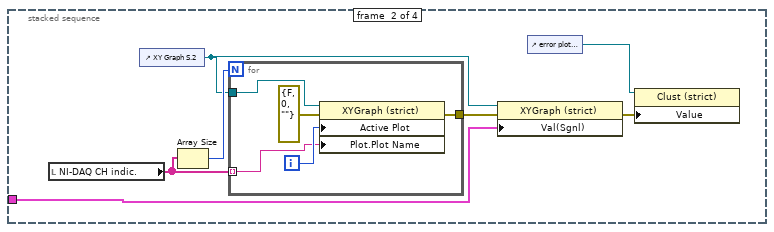
[diagram p13: hidden frame]
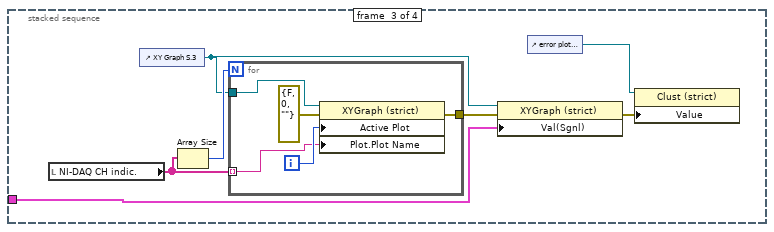
[diagram p14: hidden frame]
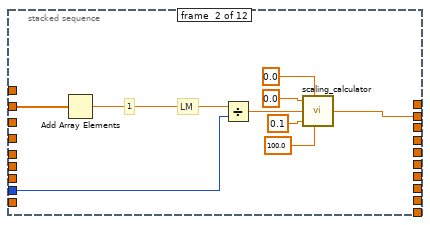
[diagram p15: hidden frame]
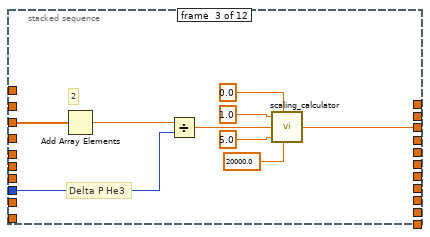
[diagram p16: hidden frame]
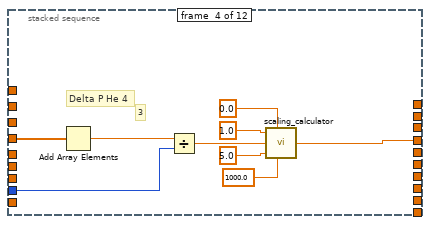
[diagram p17: hidden frame]
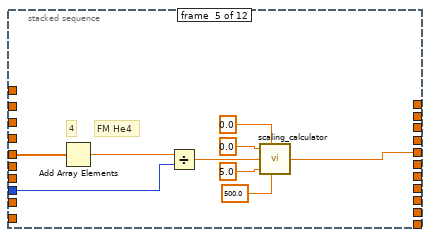
[diagram p18: hidden frame]
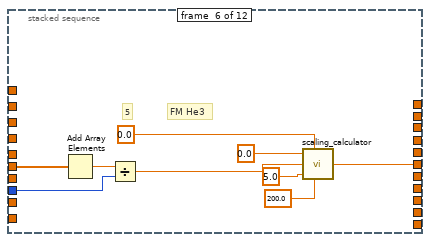
[diagram p19: hidden frame]
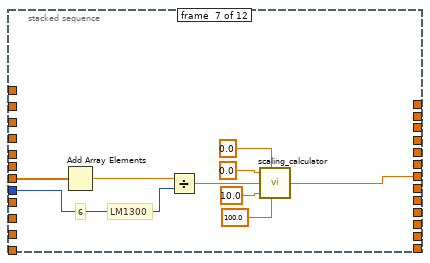
[diagram p20: hidden frame]
diagram:
  n1 = stacked-sequence {
    tunnel: [_ w146] -> w23
    tunnel: [_ w145] -> w22
    frame #0 {
      w46 = errorcluster {"status"=FALSE, "code"=0, "source"=""} ("error in")
      w41 = ".csv" ("string")
      w28 = T2."create" ("operation (0:open)")
      n2 = flat-sequence {
        frame #0 {
          w60 = i32[] [0, 1, 2, 3, 4, 5, 6, 7] ("idx in")
          # "CONSTANTS"
          "U idx" <- w60
          "D idx" <- w60
          "Q idx" <- i32[] [0, 1, 2, 3, 4, 5, 6, 7, 8, 9, 10, 11] ("Q idx 2")
          "DAQ CH OUT" <- "O1" ("DAQ CH OUT 2")
          "DAQ CH 2" <- string[] ["Q1", "Q2", "Q3", "Q4", "Q5", "Q6", "Q7", "Q8", "Q9", "Q10", "Q11", "Q12"] ("DAQ CH")
          "LSI-D CH 2" <- string[] ["D1", "D2", "D3", "D4", "D5", "D6", "D7", "D8"] ("LSI-D CH")
          "LSI-U CH 2" <- string[] ["U1", "U2", "U3", "U4", "U5", "U6", "U7", "U8"] ("LSI-U CH 3")
        }
      }
      n3 = Get Date/Time In Seconds() -> (seconds since 1Jan1904=w54:timestamp)
      n4 = Format Date/Time String(time format string (%c)="%Y%m%d_%H%M%S_", seconds (now)=w54) -> (date/time string=w32:string)  [unwired: 1 in]
      "date/time string" <- w32
      n5 = Concatenate Strings(w32, "CSV filename suffix", "_DAQ_RAW" ("string"), ".csv" ("string")) -> (w29:string)
      n6 = Concatenate Strings(w32, "CSV filename suffix", "_LSIU" ("string"), w41) -> (w51:string)
      n7 = Concatenate Strings(w32, "CSV filename suffix", "_LSID" ("string"), w41) -> (w40:string)
      n8 = Concatenate Strings(w32, "CSV filename suffix", "_DAQ" ("string"), w41) -> (w49:string)
      n9 = Build Path(base path="base path", name or relative path=w29) -> (appended path=w27:path)
      n10 = Build Path(base path="base path", name or relative path=w51) -> (appended path=w52:path)
      n11 = Build Path(base path="base path", name or relative path=w40) -> (appended path=w39:path)
      n12 = Build Path(base path="base path", name or relative path=w49) -> (appended path=w47:path)
      n13 = Open/Create/Replace File(file path (use dialog)=w52, error in=w46, operation (0:open)=w28) -> (refnum out=w45:refnum<file>)  [unwired: 3 in, 2 out]
      "ref LSI-U" <- w45
      n14 = Open/Create/Replace File(file path (use dialog)=w47, error in=w46, operation (0:open)=w28) -> (refnum out=w44:refnum<file>, error out=w38:errorcluster)  [unwired: 3 in, 1 out]
      "ref DAQ" <- w44
      n15 = Open/Create/Replace File(file path (use dialog)=w39, error in=w38, operation (0:open)=w28) -> (refnum out=w35:refnum<file>, error out=w26:errorcluster)  [unwired: 3 in, 1 out]
      "ref LSI-D" <- w35
      n16 = Open/Create/Replace File(file path (use dialog)=w27, error in=w26, operation (0:open)=w28) -> (refnum out=w24:refnum<file>, error out=w25:errorcluster)  [unwired: 3 in, 1 out]
      "ref RAW" <- w24
      n17 = flat-sequence {
        tunnel: w45 -> [w77]
        tunnel: w25 -> [w76]
        tunnel: [w72] -> w37
        tunnel: w37 -> [w82]
        tunnel: [w81] -> w36
        tunnel: w35 -> [w80]
        tunnel: w36 -> [w100]
        tunnel: w44 -> [w99]
        tunnel: [w98] -> w43
        tunnel: w24 -> [w97]
        frame #0 {
          # "Write the column names"
          n18 = local read "LSI-U CH labels"() -> (w70:string[])
          n19 = Array To Cluster(array=w70) -> (cluster=w69:T3)
          n20 = Unbundle(w69) -> ("LSI-U CH labels[0]"=w68:string, "LSI-U CH labels[1]"=w67:string, "LSI-U CH labels[2]"=w66:string, "LSI-U CH labels[3]"=w65:string, "LSI-U CH labels[4]"=w64:string, "LSI-U CH labels[5]"=w63:string, "LSI-U CH labels[6]"=w62:string, "LSI-U CH labels[7]"=w61:string)  [unwired: 1 out]
          n21 = Format Into String(format string="%s,%s,%s,%s,%s,%s,%s,%s,%s,%s,%s,%s\\n" ("time format string (%c)"), initial string=w77, error in=w76, "INDEX" ("input 1"), "Datetime" ("input 1"), "UNIX_time" ("input 1"), "LV_time" ("input 1"), w68, w67, w66, w65, w64, w63, w62, w61) -> (error out=w72:errorcluster)  [unwired: 1 out]
        }
        frame #1 {
          # "Write the column names"
          n22 = local read "LSI-D CH labels"() -> (w87:string[])
          n23 = Array To Cluster(array=w87) -> (cluster=w88:T4)
          n24 = Unbundle(w88) -> ("LSI-D CH labels[0]"=w89:string, "LSI-D CH labels[1]"=w90:string, "LSI-D CH labels[2]"=w91:string, "LSI-D CH labels[3]"=w92:string, "LSI-D CH labels[4]"=w93:string, "LSI-D CH labels[5]"=w94:string, "LSI-D CH labels[6]"=w95:string, "LSI-D CH labels[7]"=w96:string)  [unwired: 1 out]
          n25 = Format Into String(format string="%s,%s,%s,%s,%s,%s,%s,%s,%s,%s,%s,%s\\n" ("time format string (%c)"), initial string=w80, error in=w82, "INDEX" ("input 1"), "Datetime" ("input 1"), "UNIX_time" ("input 1"), "LV_time" ("input 1"), w89, w90, w91, w92, w93, w94, w95, w96) -> (error out=w81:errorcluster)  [unwired: 1 out]
        }
        frame #2 {
          n26 = stacked-sequence {
            tunnel: w100 -> [w117 w137]
            tunnel: w99 -> [w116 _]
            tunnel: [w115 _] -> w98
            tunnel: w97 -> [_ w123]
            frame #0 {
              # "Write the column names"
              n27 = local read "NI DAQ AIN labels"() -> (w113:string[])
              n28 = Index Array(array=w113) -> (element #1=w112:string, element #2=w111:string, element #3=w110:string, element #4=w109:string, element #5=w107:string, element #6=w108:string, element #7=w106:string, element #8=w105:string, element #9=w104:string, element #10=w103:string, element #11=w102:string, element #12=w101:string)  [unwired: 13 in, 1 out]
              n29 = Format Into String(format string="%s,%s,%s,%s,%s,%s,%s,%s,%s,%s,%s,%s,%s,%s,%s,%s\\n" ("time format string (%c)"), initial string=w116, error in=w117, "INDEX" ("input 1"), "Datetime" ("input 1"), "UNIX_time" ("input 1"), "LV_time" ("input 1"), w112, w111, w110, w109, w107, w108, w106, w105, w104, w103, w102, w101) -> (error out=w115:errorcluster)  [unwired: 1 out]
            }
            frame #1 {
              # "Write the column names"
              n30 = local read "NI DAQ AIN labels"() -> (w135:string[])
              n31 = Index Array(array=w135) -> (element #1=w134:string, element #2=w133:string, element #3=w132:string, element #4=w131:string, element #5=w129:string, element #6=w130:string, element #7=w128:string, element #8=w127:string, element #9=w126:string, element #10=w125:string, element #11=w124:string, element #12=w122:string)  [unwired: 12 in]
              n32 = Format Into String(format string="%s,%s,%s,%s,%s,%s,%s,%s,%s,%s,%s,%s,%s,%s,%s,%s\\n" ("time format string (%c)"), initial string=w123, error in=w137, "INDEX" ("input 1"), "Datetime" ("input 1"), "UNIX_time" ("input 1"), "LV_time" ("input 1"), w134, w133, w132, w131, w129, w130, w128, w127, w126, w125, w124, w122) -> ()  [unwired: 2 out]
            }
          }
        }
      }
      "error out\n(file creation)" <- w43
    }
    frame #1 {
      # "DAQ config"
      n33 = feedback #1() -> (w142:errorcluster)  [unwired: 1 in]
      n34 = stacked-sequence {
        tunnel: [w147 _] -> w143
        tunnel: [w148 _] -> w146
        tunnel: [_ w176] -> w145
        tunnel: [_ w175] -> w144
        tunnel: w142 -> [_ w168]
        frame #0 {
          # "read task"
          n35 = local read "date/time string"() -> (w158:string)
          n36 = Concatenate Strings(w158, "AI" ("new task name")) -> (w156:string)
          n37 = call <vilib>:"DAQmx Create Task.vi"("new task name"=w156, "error in"=errorcluster {"status"=FALSE, "code"=0, "source"=""}) -> ("task out"=w154:refnum<k21>, "error out"=w155:errorcluster)  [unwired: 12 in]
          n38 = for {
            shift-right: [w167] -> w149
            shift-left: w155 -> [w166]
            shift-right: [w165] -> w150
            shift-left: w154 -> [w164]
            tunnel: "DAQ analog channels" -> [w163] mode=indexing
            tunnel: "V_min(in)" -> [w162] mode=indexing
            tunnel: "V_max(in)" -> [w161] mode=indexing
            w160 = 10106 items=["Default"=-1, "RSE"=10083, "NRSE"=10078, "Differential"=10106, "Pseudodifferential"=12529] ("input terminal configuration")
            n39 = call-poly <vilib>:"DAQmx Create Virtual Channel.vi"("task in"=w164, "maximum value"=w161, "minimum value"=w162, "input terminal configuration"=w160, "physical channels"=w163, "error in"=w166) -> ("task out"=w165:refnum<k21>, "error out"=w167:errorcluster)  [unwired: 8 in]
          }
          n40 = call <vilib>:"DAQmx Start Task.vi"("task/channels in"=w150, "error in"=w149) -> ("task out"=w148:refnum<k21>, "error out"=w147:errorcluster)  [unwired: 12 in]
        }
        frame #1 {
          # "write task"
          n41 = local read "date/time string"() -> (w171:string)
          n42 = Concatenate Strings(w171, "AO" ("new task name")) -> (w169:string)
          n43 = call <vilib>:"DAQmx Create Task.vi"("new task name"=w169, "error in"=w168) -> ("task out"=w173:refnum<k21>, "error out"=w172:errorcluster)  [unwired: 12 in]
          n44 = case shown="True" "DAQ OUT ON?" {
            tunnel: [w178 w185] -> w176
            tunnel: [w177 w184] -> w175
            tunnel: w173 -> [w178 w183]
            tunnel: w172 -> [w177 w182]
            frame False {
            }
            frame True {
              w187 = -1 items=["Default"=-1, "RSE"=10083, "Differential"=10106, "Pseudodifferential"=12529] ("output terminal configuration")
              w186 = 10348 items=["Volts"=10348, "From Custom Scale"=10065] ("units")
              n45 = call-poly <vilib>:"DAQmx Create Virtual Channel.vi"("task in"=w183, "maximum value"="V_max(out)", "minimum value"="V_min(out)", "output terminal configuration"=w187, "physical channels"="DAQ  OUT", "units"=w186, "error in"=w182) -> ("task out"=w189:refnum<k21>, "error out"=w188:errorcluster)  [unwired: 7 in]
              n46 = call <vilib>:"DAQmx Start Task.vi"("task/channels in"=w189, "error in"=w188) -> ("task out"=w185:refnum<k21>, "error out"=w184:errorcluster)  [unwired: 12 in]
            }
          }
        }
      }
      "error out\n(DAQ config)" <- w144
      n47 = feedback-in #1(w143) -> ()
    }
  }
  n48 = while {
    stop <- w190 stop-if-true
    n49 = flat-sequence {
      frame #0 {
      }
    }
    n50 = event shown="[1] \"log/linear 1\": Value Change" {
      selector: _ -> [_ _ _ _ _ _]
      dyn-events: _ -> [_ _ _ _ _ _]
      timeout: _ -> [_ _ _ _ _ _]
      tunnel: [_ _ _ _ _ TRUE ("stop")] -> w190
      event Timeout {
        n51 = event-data() -> ()  [unwired: 1 in, 3 out]
      }
      event "log/linear 1": Value Change {
        n52 = event-data() -> ()  [unwired: 1 in, 6 out]
        n53 = flat-sequence {
          frame #0 {
            n54 = local read "log/linear 1"() -> (w196:bool)
            n55 = control-ref of="XY Graph S.1"() -> (w192:refnum<vi>)
            n56 = Boolean To (0,1)(Boolean=w196) -> (0, 1=w195:i16)
            n57 = property class="XYGraph (strict)"(reference=w192, error in=errorcluster {"status"=FALSE, "code"=0, "source"=""} ("error in (no error)"), "YScale.Mapping Mode"=w195) -> (error out=w193:errorcluster)  [unwired: 1 out]
            n58 = control-ref of="error plot cosmetic 2"() -> (w194:refnum<vi>)
            n59 = property class="Clust (strict)"(reference=w194, "Value"=w193) -> ()  [unwired: 1 in, 2 out]
          }
        }
      }
      event "log/linear 2": Value Change {
        n60 = event-data() -> ()  [unwired: 1 in, 6 out]
        n61 = flat-sequence {
          frame #0 {
            n62 = local read "log/linear 2"() -> (w202:bool)
            n63 = control-ref of="XY Graph S.2"() -> (w198:refnum<vi>)
            n64 = Boolean To (0,1)(Boolean=w202) -> (0, 1=w201:i16)
            n65 = property class="XYGraph (strict)"(reference=w198, error in=errorcluster {"status"=FALSE, "code"=0, "source"=""} ("error in (no error)"), "YScale.Mapping Mode"=w201) -> (error out=w199:errorcluster)  [unwired: 1 out]
            n66 = control-ref of="error plot cosmetic 2"() -> (w200:refnum<vi>)
            n67 = property class="Clust (strict)"(reference=w200, "Value"=w199) -> ()  [unwired: 1 in, 2 out]
          }
        }
      }
      event "log/linear 3": Value Change {
        n68 = event-data() -> ()  [unwired: 1 in, 6 out]
        n69 = flat-sequence {
          frame #0 {
            n70 = local read "log/linear 3"() -> (w205:bool)
            n71 = control-ref of="XY Graph S.3"() -> (w204:refnum<vi>)
            n72 = Boolean To (0,1)(Boolean=w205) -> (0, 1=w208:i16)
            n73 = property class="XYGraph (strict)"(reference=w204, error in=errorcluster {"status"=FALSE, "code"=0, "source"=""} ("error in (no error)"), "YScale.Mapping Mode"=w208) -> (error out=w206:errorcluster)  [unwired: 1 out]
            n74 = control-ref of="error plot cosmetic 2"() -> (w207:refnum<vi>)
            n75 = property class="Clust (strict)"(reference=w207, "Value"=w206) -> ()  [unwired: 1 in, 2 out]
          }
        }
      }
      event "log/linear 4": Value Change {
        n76 = event-data() -> ()  [unwired: 1 in, 6 out]
        n77 = flat-sequence {
          frame #0 {
            n78 = local read "log/linear 4"() -> (w211:bool)
            n79 = control-ref of="XY Graph S.4"() -> (w210:refnum<vi>)
            n80 = Boolean To (0,1)(Boolean=w211) -> (0, 1=w214:i16)
            n81 = property class="XYGraph (strict)"(reference=w210, error in=errorcluster {"status"=FALSE, "code"=0, "source"=""} ("error in (no error)"), "YScale.Mapping Mode"=w214) -> (error out=w212:errorcluster)  [unwired: 1 out]
            n82 = control-ref of="error plot cosmetic 2"() -> (w213:refnum<vi>)
            n83 = property class="Clust (strict)"(reference=w213, "Value"=w212) -> ()  [unwired: 1 in, 2 out]
          }
        }
      }
      event "stop": Value Change {
        n84 = event-data() -> ()  [unwired: 1 in, 6 out]
      }
    }
    n85 = Wait (ms)(milliseconds to wait=u32 500) -> ()  [unwired: 1 out]
  }
  n86 = call "Initialize.vi"("VISA resource name"="VISA LSI218 UP", "error in (no error)"=errorcluster {"status"=FALSE, "code"=0, "source"=""}) -> ("VISA resource name out"=w4:refnum<visa-resource-name>, "error out"=w3:errorcluster)  [unwired: 12 in]
  n87 = call "Initialize.vi"("VISA resource name"="VISA LSI218 DOWN", "error in (no error)"=errorcluster {"status"=FALSE, "code"=0, "source"=""}) -> ("VISA resource name out"=w6:refnum<visa-resource-name>, "error out"=w5:errorcluster)  [unwired: 12 in]
  n88 = while {
    shift-right: [w232] -> _
    shift-left: dbl[] [] -> [w243]
    shift-right: [w235] -> _
    shift-left: dbl[][] [] -> [w236]
    tunnel: w23 -> [w239]
    tunnel: w22 -> [w238]
    shift-right: [w231] -> _
    shift-left: dbl[][] [] -> [w237]
    tunnel: [w227] -> w12
    tunnel: [w226] -> w11
    tunnel: [w225] -> w10
    tunnel: w6 -> [w224]
    tunnel: w5 -> [w223]
    tunnel: w4 -> [w222]
    tunnel: w3 -> [w221]
    shift-right: [w218] -> _
    shift-left: dbl[][] [] -> [w217]
    i -> [w240]
    stop <- "stop" stop-if-true
    n89 = Get Date/Time In Seconds() -> (seconds since 1Jan1904=→"current time":timestamp)
    n90 = local read "current time"() -> (w241:timestamp)
    n91 = Multiply(x="Wait (s)", y=1000) -> (x*y=w228:i32)
    n92 = To Double Precision Float(number=w241) -> (double precision float=w242:dbl)
    n93 = Wait (ms)(milliseconds to wait=w228) -> ()  [unwired: 1 out]
    n94 = Build Array (concatenate)(w243, w242) -> (w232:dbl[])
    n95 = flat-sequence {
      tunnel: w232 -> [w576]
      tunnel: w236 -> [w652]
      tunnel: [w642] -> w233
      tunnel: w224 -> [w648]
      tunnel: w223 -> [w647]
      tunnel: w222 -> [w646]
      tunnel: w221 -> [w645]
      tunnel: [w577] -> w219
      tunnel: w217 -> [w578]
      tunnel: [w698] -> w234
      tunnel: w233 -> [w698]
      tunnel: [w697] -> w220
      tunnel: w219 -> [w697]
      tunnel: [w723] -> w235
      tunnel: w234 -> [w723]
      tunnel: [w718] -> w218
      tunnel: w220 -> [w718]
      frame #0 {
        n96 = local read "LSI-U CH labels"() -> (→"LSI-U CH indic,":string[])
        n97 = local read "LSI-D CH labels"() -> (→"LSI-D CH indic.":string[])
        n98 = call "Data Sensor.vi"("VISA resource name"=w648, "error in (no error)"=w647) -> ("Input 1"=w614:dbl, "Input 2"=w613:dbl, "Input 3"=w612:dbl, "VISA resource name out"=w650:refnum<visa-resource-name>, "Input 4"=w611:dbl, "Input 5"=w610:dbl, "Input 6"=w609:dbl, "Input 8"=w607:dbl, "Input 7"=w608:dbl, "error out"=w649:errorcluster)  [unwired: 4 in]
        n99 = call "Data Sensor.vi"("VISA resource name"=w646, "error in (no error)"=w645) -> ("Input 1"=w662:dbl, "Input 2"=w661:dbl, "Input 3"=w660:dbl, "VISA resource name out"=w654:refnum<visa-resource-name>, "Input 4"=w644:dbl, "Input 5"=w659:dbl, "Input 6"=w658:dbl, "Input 8"=w656:dbl, "Input 7"=w657:dbl, "error out"=w655:errorcluster)  [unwired: 4 in]
        n100 = call "Close.vi"("VISA resource name"=w650, "error in (no error)"=w649) -> ("error out"=→"error out \n(LSID)":errorcluster)  [unwired: 13 in]
        n101 = call "Close.vi"("VISA resource name"=w654, "error in (no error)"=w655) -> ("error out"=→"error out \n(LSIU)":errorcluster)  [unwired: 13 in]
        n102 = Build Array(w614, w613, w612, w611, w610, w609, w608, w607) -> (w571:dbl[])
        "LSI-D out" <- w571
        "LSI-D out 1" <- w571
        "LSI-D out 2" <- w571
        n103 = Build Array(w662, w661, w660, w644, w659, w658, w657, w656) -> (w573:dbl[])
        "LSI-U out" <- w573
        "LSI-U out 1" <- w573
        "LSI-U out 2" <- w573
        n104 = Array Size(array=w573) -> ()  [unwired: 1 out]
        n105 = Build Array (concatenate)(w578, w571) -> (w577:dbl[][])
        n106 = Build Array (concatenate)(w652, w573) -> (w642:dbl[][])
        n107 = Index Array(array=w577, index (col) #1=0 ("disabled index (col)"), index (col) #2=1 ("index (col)"), index (col) #3=2 ("index (col)"), index (col) #4=3 ("index (col)"), index (col) #5=4 ("index (col)"), index (col) #6=5 ("index (col)"), index (col) #7=6 ("index (col)"), index (col) #8=7 ("index (col)"), index (col) #9=8 ("index (col)")) -> (element #1=w580:dbl[], element #2=w589:dbl[], element #3=w590:dbl[], element #4=w591:dbl[], element #5=w592:dbl[], element #6=w593:dbl[], element #7=w594:dbl[], element #8=w595:dbl[], element #9=w596:dbl[])  [unwired: 9 in]
        n108 = Index Array(array=w642, index (col) #1=0 ("disabled index (col)"), index (col) #2=1 ("index (col)"), index (col) #3=2 ("index (col)"), index (col) #4=3 ("index (col)"), index (col) #5=4 ("index (col)"), index (col) #6=5 ("index (col)"), index (col) #7=6 ("index (col)"), index (col) #8=7 ("index (col)"), index (col) #9=8 ("index (col)")) -> (element #1=w640:dbl[], element #2=w631:dbl[], element #3=w630:dbl[], element #4=w629:dbl[], element #5=w628:dbl[], element #6=w627:dbl[], element #7=w626:dbl[], element #8=w625:dbl[], element #9=w624:dbl[])  [unwired: 9 in]
        n109 = Bundle(w576, w580) -> (w597:cluster{dbl[], dbl[]})  [unwired: 1 in]
        n110 = Bundle(w576, w589) -> (w598:cluster{dbl[], dbl[]})  [unwired: 1 in]
        n111 = Bundle(w576, w590) -> (w599:cluster{dbl[], dbl[]})  [unwired: 1 in]
        n112 = Bundle(w576, w591) -> (w600:cluster{dbl[], dbl[]})  [unwired: 1 in]
        n113 = Bundle(w576, w592) -> (w601:cluster{dbl[], dbl[]})  [unwired: 1 in]
        n114 = Bundle(w576, w593) -> (w602:cluster{dbl[], dbl[]})  [unwired: 1 in]
        n115 = Bundle(w576, w594) -> (w603:cluster{dbl[], dbl[]})  [unwired: 1 in]
        n116 = Bundle(w576, w595) -> (w604:cluster{dbl[], dbl[]})  [unwired: 1 in]
        n117 = Bundle(w576, w596) -> (w605:cluster{dbl[], dbl[]})  [unwired: 1 in]
        n118 = Bundle(w576, w640) -> (w623:cluster{dbl[], dbl[]})  [unwired: 1 in]
        n119 = Bundle(w576, w631) -> (w622:cluster{dbl[], dbl[]})  [unwired: 1 in]
        n120 = Bundle(w576, w630) -> (w621:cluster{dbl[], dbl[]})  [unwired: 1 in]
        n121 = Bundle(w576, w629) -> (w620:cluster{dbl[], dbl[]})  [unwired: 1 in]
        n122 = Bundle(w576, w628) -> (w619:cluster{dbl[], dbl[]})  [unwired: 1 in]
        n123 = Bundle(w576, w627) -> (w618:cluster{dbl[], dbl[]})  [unwired: 1 in]
        n124 = Bundle(w576, w626) -> (w617:cluster{dbl[], dbl[]})  [unwired: 1 in]
        n125 = Bundle(w576, w625) -> (w616:cluster{dbl[], dbl[]})  [unwired: 1 in]
        n126 = Bundle(w576, w624) -> (w615:cluster{dbl[], dbl[]})  [unwired: 1 in]
        n127 = Build Array(w597, w598, w599, w600, w601, w602, w603, w604, w605) -> (→"Graph LSI-D 1" →"Graph LSI-D 2":cluster{dbl[], dbl[]}[])
        n128 = Build Array(w623, w622, w621, w620, w619, w618, w617, w616, w615) -> (→"Graph LSI-U 1" →"Graph LSI-U 2":cluster{dbl[], dbl[]}[])
        n129 = feedback #2() -> (w565:errorcluster)  [unwired: 1 in]
        n130 = stacked-sequence {
          tunnel: [w663 _] -> w566
          tunnel: [_ w672] -> w564
          tunnel: w565 -> [_ w671]
          frame #0 {
            n131 = local read "LSI-D CH indic."() -> (w664:string[])
            n132 = Array Size(array=w664) -> (size(s)=w665:i32)
            n133 = for {
              N: w665 -> [_]
              tunnel: w664 -> [w668] mode=indexing
              tunnel: [w667] -> w663
              i -> [w669]
              n134 = control-ref of="Graph LSI-D 1"() -> (w666:refnum<vi>)
              n135 = property class="XYGraph (strict)"(reference=w666, error in=errorcluster {"status"=FALSE, "code"=0, "source"=""} ("error in (no error)"), "Active Plot"=w669, "Plot.Plot Name"=w668) -> (error out=w667:errorcluster)  [unwired: 1 out]
            }
          }
          frame #1 {
            n136 = local read "LSI-D CH indic."() -> (w673:string[])
            n137 = Array Size(array=w673) -> (size(s)=w674:i32)
            n138 = for {
              N: w674 -> [_]
              tunnel: w673 -> [w678] mode=indexing
              tunnel: [w677] -> w672
              tunnel: w671 -> [w676]
              i -> [w679]
              n139 = control-ref of="Graph LSI-D 2"() -> (w675:refnum<vi>)
              n140 = property class="XYGraph (strict)"(reference=w675, error in=w676, "Active Plot"=w679, "Plot.Plot Name"=w678) -> (error out=w677:errorcluster)  [unwired: 1 out]
            }
          }
        }
        n141 = feedback-in #2(w566) -> ()
        n142 = feedback #3() -> (w569:errorcluster)  [unwired: 1 in]
        n143 = stacked-sequence {
          tunnel: [w680 _] -> w570
          tunnel: w569 -> [_ w689]
          tunnel: [_ w688] -> w568
          frame #0 {
            n144 = local read "LSI-U CH indic,"() -> (w681:string[])
            n145 = Array Size(array=w681) -> (size(s)=w682:i32)
            n146 = for {
              N: w682 -> [_]
              tunnel: w681 -> [w684] mode=indexing
              tunnel: [w683] -> w680
              i -> [w685]
              n147 = control-ref of="Graph LSI-U 1"() -> (w687:refnum<vi>)
              n148 = property class="XYGraph (strict)"(reference=w687, error in=errorcluster {"status"=FALSE, "code"=0, "source"=""} ("error in (no error)"), "Active Plot"=w685, "Plot.Plot Name"=w684) -> (error out=w683:errorcluster)  [unwired: 1 out]
            }
          }
          frame #1 {
            n149 = local read "LSI-U CH indic,"() -> (w690:string[])
            n150 = Array Size(array=w690) -> (size(s)=w691:i32)
            n151 = for {
              N: w691 -> [_]
              tunnel: w690 -> [w695] mode=indexing
              tunnel: w689 -> [w694]
              tunnel: [w693] -> w688
              i -> [w696]
              n152 = control-ref of="Graph LSI-U 2"() -> (w692:refnum<vi>)
              n153 = property class="XYGraph (strict)"(reference=w692, error in=w694, "Active Plot"=w696, "Plot.Plot Name"=w695) -> (error out=w693:errorcluster)  [unwired: 1 out]
            }
          }
        }
        n154 = feedback-in #3(w570) -> ()
        n155 = control-ref of="error plot content"() -> (w575:refnum<vi>)
        n156 = control-ref of="error plot content"() -> (w574:refnum<vi>)
        n157 = property class="Clust (strict)"(reference=w575, "Value"=w564) -> ()  [unwired: 1 in, 2 out]
        n158 = property class="Clust (strict)"(reference=w574, "Value"=w568) -> ()  [unwired: 1 in, 2 out]
      }
      frame #1 {
      }
      frame #2 {
        n159 = local read "LSI-D out"() -> (w699:dbl[])
        n160 = local read "LSI-U out"() -> (w734:dbl[])
        n161 = local read "current time"() -> (w714:timestamp)
        n162 = local read "current time"() -> (w722:timestamp)
        n163 = Array To Cluster(array=w699) -> (cluster=w704:T5)
        n164 = Array To Cluster(array=w734) -> (cluster=w733:T6)
        n165 = To Double Precision Float(number=w714) -> (double precision float=w702:dbl)
        n166 = To Double Precision Float(number=w722) -> (double precision float=w736:dbl)
        n167 = call "LV_UNIX.vi"("current time"=w714) -> ("date/time string"=w716:string, "UNIX time (s)"=w715:dbl)  [unwired: 9 in]
        n168 = Unbundle(w704) -> ("LSI-D out[0]"=w705:dbl, "LSI-D out[1]"=w706:dbl, "LSI-D out[2]"=w707:dbl, "LSI-D out[3]"=w708:dbl, "LSI-D out[4]"=w709:dbl, "LSI-D out[5]"=w710:dbl, "LSI-D out[6]"=w711:dbl, "LSI-D out[7]"=w712:dbl)  [unwired: 1 out]
        n169 = call "LV_UNIX.vi"("current time"=w722) -> ("date/time string"=w720:string, "UNIX time (s)"=w721:dbl)  [unwired: 9 in]
        n170 = Unbundle(w733) -> ("LSI-U out[0]"=w732:dbl, "LSI-U out[1]"=w731:dbl, "LSI-U out[2]"=w730:dbl, "LSI-U out[3]"=w729:dbl, "LSI-U out[4]"=w728:dbl, "LSI-U out[5]"=w727:dbl, "LSI-U out[6]"=w726:dbl, "LSI-U out[7]"=w725:dbl)  [unwired: 1 out]
        n171 = local read "error out\n(file creation)"() -> (w701:errorcluster)
        n172 = local read "error out\n(file creation)"() -> (w737:errorcluster)
        n173 = local read "ref LSI-D"() -> (w700:refnum<file>)
        n174 = local read "ref LSI-U"() -> (w738:refnum<file>)
        n175 = local read "Cycle #"() -> (w717:i32)
        n176 = local read "Cycle #"() -> (w719:i32)
        n177 = Format Into String(format string="%d,%s,%10.4f,%10.4f,%5.6f,%5.6f,%5.6f,%5.6f,%5.6f,%5.6f,%5.6f,%5.6f\\n", initial string=w700, error in=w701, w717, w716, w715, w702, w705, w706, w707, w708, w709, w710, w711, w712) -> (error out=→"error out \n(record LSID)":errorcluster)  [unwired: 1 out]
        n178 = Format Into String(format string="%d,%s,%10.4f,%10.4f,%5.6f,%5.6f,%5.6f,%5.6f,%5.6f,%5.6f,%5.6f,%5.6f\\n", initial string=w738, error in=w737, w719, w720, w721, w736, w732, w731, w730, w729, w728, w727, w726, w725) -> (error out=→"error out \n(record LSIU)":errorcluster)  [unwired: 1 out]
      }
    }
    n179 = stacked-sequence {
      tunnel: w239 -> [w357 _]
      tunnel: w238 -> [_ w554]
      tunnel: [_ w552] -> w226
      tunnel: w237 -> [w339 _]
      tunnel: [w310 _] -> w231
      tunnel: w232 -> [w251 _]
      tunnel: [w338 _] -> w227
      tunnel: [_ w550] -> w225
      frame #0 {
        n180 = local read "error out\n(DAQ config)"() -> (w353:errorcluster)
        n181 = local read "NI DAQ AIN labels"() -> (→"NI-DAQ CH indic.":string[])
        n182 = local read "DAQ sample #"() -> (w334:i32)
        n183 = call <vilib>:"DAQmx Read (Analog 2D DBL NChan NSamp).vi"("task/channels in"=w357, "number of samples per channel"=w334, "timeout"=100.0, "error in"=w353) -> ("task out"=w338:refnum<k21>, "data"=w287:dbl[][], "error out"=→"error out \n(DAQ IN)":errorcluster)  [unwired: 9 in]
        n184 = Index Array(array=w287, index (col)=0 ("disabled index (col)")) -> (element=→"RAW (V)":dbl[])  [unwired: 1 in]
        n185 = Index Array(array=w287, index (row) #1=0 ("index (row)"), index (row) #2=1 ("index (row)"), index (row) #3=2 ("index (row)"), index (row) #4=3 ("index (row)"), index (row) #5=4 ("disabled index (col)"), index (row) #6=5 ("index (col)"), index (row) #7=6 ("disabled index (row)"), index (row) #8=7 ("disabled index (row)"), index (row) #9=8 ("disabled index (row)"), index (row) #10=9 ("index (row)"), index (row) #11=10 ("index (row)"), index (row) #12=11 ("index (row)")) -> (element #1=w319:dbl[], element #2=w324:dbl[], element #3=w327:dbl[], element #4=w321:dbl[], element #5=w320:dbl[], element #6=w318:dbl[], element #7=w314:dbl[], element #8=w313:dbl[], element #9=w312:dbl[], element #10=w289:dbl[], element #11=w288:dbl[], element #12=w248:dbl[])  [unwired: 12 in]
        n186 = stacked-sequence {
          tunnel: [w445 _ _ _ _ _ _ _ _ _ _ _] -> w337
          tunnel: [_ w454 _ _ _ _ _ _ _ _ _ _] -> w335
          tunnel: w334 -> [w443 w450 w459 w468 w477 w486 w496 w504 w515 w526 w538 w549]
          tunnel: [_ _ w461 _ _ _ _ _ _ _ _ _] -> w333
          tunnel: w324 -> [_ w451 _ _ _ _ _ _ _ _ _ _]
          tunnel: [_ _ _ w470 _ _ _ _ _ _ _ _] -> w330
          tunnel: [_ _ _ _ w479 _ _ _ _ _ _ _] -> w329
          tunnel: [_ _ _ _ _ w488 _ _ _ _ _ _] -> w328
          tunnel: w327 -> [_ _ w460 _ _ _ _ _ _ _ _ _]
          tunnel: [_ _ _ _ _ _ w495 _ _ _ _ _] -> w326
          tunnel: w321 -> [_ _ _ w469 _ _ _ _ _ _ _ _]
          tunnel: w320 -> [_ _ _ _ w478 _ _ _ _ _ _ _]
          tunnel: w319 -> [w441 _ _ _ _ _ _ _ _ _ _ _]
          tunnel: w318 -> [_ _ _ _ _ w487 _ _ _ _ _ _]
          tunnel: w314 -> [_ _ _ _ _ _ w497 _ _ _ _ _]
          tunnel: w313 -> [_ _ _ _ _ _ _ w506 _ _ _ _]
          tunnel: w312 -> [_ _ _ _ _ _ _ _ w513 _ _ _]
          tunnel: [_ _ _ _ _ _ _ w505 _ _ _ _] -> w311
          tunnel: w289 -> [_ _ _ _ _ _ _ _ _ w524 _ _]
          tunnel: w288 -> [_ _ _ _ _ _ _ _ _ _ w534 _]
          tunnel: [_ _ _ _ _ _ _ _ _ _ _ w548] -> w258
          tunnel: [_ _ _ _ _ _ _ _ _ w525 _ _] -> w256
          tunnel: [_ _ _ _ _ _ _ _ _ _ w537 _] -> w257
          tunnel: [_ _ _ _ _ _ _ _ _ _ _ w545] -> w261
          tunnel: [_ _ _ _ _ _ _ _ _ w523 _ _] -> w262
          tunnel: [_ _ _ _ _ _ _ _ _ _ w535 _] -> w265
          tunnel: [_ _ _ _ _ _ _ _ _ _ w535 _] -> w264
          tunnel: [_ _ _ _ _ _ _ _ w514 _ _ _] -> w255
          tunnel: w248 -> [_ _ _ _ _ _ _ _ _ _ _ w544]
          frame #0 {
            # "0"
            # "P (4K)"
            n187 = Add Array Elements(numeric array=w441) -> (sum=w444:dbl)
            n188 = Divide(x=w444, y=w443) -> (x/y=w442:dbl)
            n189 = call "scaling_calculator.vi"("x1"=1.0, "y1"=0.0 ("x1"), "x"=w442, "x2"=3.0 ("x1"), "y2"=100000.0 ("x1")) -> ("y"=w445:dbl)  [unwired: 2 in]
          }
          frame #1 {
            # "1"
            # "LM"
            n190 = Add Array Elements(numeric array=w451) -> (sum=w453:dbl)
            n191 = Divide(x=w453, y=w450) -> (x/y=w452:dbl)
            n192 = call "scaling_calculator.vi"("x1"=0.0, "y1"=0.0 ("x1"), "x"=w452, "x2"=0.1 ("x1"), "y2"=100.0 ("x1")) -> ("y"=w454:dbl)  [unwired: 2 in]
          }
          frame #2 {
            # "2"
            # "Delta P He3"
            n193 = Add Array Elements(numeric array=w460) -> (sum=w463:dbl)
            n194 = Divide(x=w463, y=w459) -> (x/y=w462:dbl)
            n195 = call "scaling_calculator.vi"("x1"=1.0, "y1"=0.0 ("x1"), "x"=w462, "x2"=5.0 ("x1"), "y2"=20000.0 ("x1")) -> ("y"=w461:dbl)  [unwired: 2 in]
          }
          frame #3 {
            # "3"
            # "Delta P He 4"
            n196 = Add Array Elements(numeric array=w469) -> (sum=w472:dbl)
            n197 = Divide(x=w472, y=w468) -> (x/y=w471:dbl)
            n198 = call "scaling_calculator.vi"("x1"=1.0, "y1"=0.0 ("x1"), "x"=w471, "x2"=5.0 ("x1"), "y2"=1000.0 ("x1")) -> ("y"=w470:dbl)  [unwired: 2 in]
          }
          frame #4 {
            # "4"
            # "FM He4"
            n199 = Add Array Elements(numeric array=w478) -> (sum=w481:dbl)
            n200 = Divide(x=w481, y=w477) -> (x/y=w480:dbl)
            n201 = call "scaling_calculator.vi"("x1"=0.0, "y1"=0.0 ("x1"), "x"=w480, "x2"=5.0 ("x1"), "y2"=500.0 ("x1")) -> ("y"=w479:dbl)  [unwired: 2 in]
          }
          frame #5 {
            # "5"
            # "FM He3"
            n202 = Add Array Elements(numeric array=w487) -> (sum=w490:dbl)
            n203 = Divide(x=w490, y=w486) -> (x/y=w489:dbl)
            n204 = call "scaling_calculator.vi"("x1"=0.0, "y1"=0.0 ("x1"), "x"=w489, "x2"=5.0 ("x1"), "y2"=200.0 ("x1")) -> ("y"=w488:dbl)  [unwired: 2 in]
          }
          frame #6 {
            # "LM1300"
            # "6"
            n205 = Add Array Elements(numeric array=w497) -> (sum=w503:dbl)
            n206 = Divide(x=w503, y=w496) -> (x/y=w502:dbl)
            n207 = call "scaling_calculator.vi"("x1"=0.0, "y1"=0.0 ("x1"), "x"=w502, "x2"=10.0 ("x1"), "y2"=100.0 ("x1")) -> ("y"=w495:dbl)  [unwired: 2 in]
          }
          frame #7 {
            # "7"
            # "AI16 absolute pressure"
            n208 = Add Array Elements(numeric array=w506) -> (sum=w512:dbl)
            n209 = Divide(x=w512, y=w504) -> (x/y=w507:dbl)
            n210 = call "scaling_calculator.vi"("x1"=1.0, "y1"=0.0 ("x1"), "x"=w507, "x2"=5.0 ("x1"), "y2"=200000.0 ("x1")) -> ("y"=w505:dbl)  [unwired: 2 in]
          }
          frame #8 {
            # "8"
            # "AI17 absolute pressure"
            n211 = Add Array Elements(numeric array=w513) -> (sum=w521:dbl)
            n212 = Divide(x=w521, y=w515) -> (x/y=w516:dbl)
            n213 = call "scaling_calculator.vi"("x1"=1.0, "y1"=0.0 ("x1"), "x"=w516, "x2"=5.0 ("x1"), "y2"=200000.0 ("x1")) -> ("y"=w514:dbl)  [unwired: 2 in]
          }
          frame #9 {
            # "9"
            # "AIN18 baratron front"
            n214 = Add Array Elements(numeric array=w524) -> (sum=w527:dbl)
            n215 = Divide(x=w527, y=w526) -> (x/y=w523:dbl)
            n216 = case shown="False" TRUE {
              tunnel: [w530 w531] -> w525
              tunnel: w523 -> [w529 w532]
              frame False {
                n217 = call "scaling_calculator_baratron.vi"("x"=w529, "offset subt"="Bar_anal Vbar offset") -> ("y (Pa)"=w530:dbl)  [unwired: 4 in, 1 out]
              }
              frame True {
                n218 = call "baratron_conv_analog.vi"("V_ana (V)"=w532) -> ("y (Pa)"=w531:dbl)  [unwired: 10 in]
              }
            }
          }
          frame #10 {
            # "10"
            # "AIN 19 baratron buffer 1"
            n219 = Add Array Elements(numeric array=w534) -> (sum=w536:dbl)
            n220 = Divide(x=w536, y=w538) -> (x/y=w535:dbl)
            n221 = case shown="False" TRUE {
              tunnel: [w541 w542] -> w537
              tunnel: w535 -> [w539 w543]
              frame False {
                n222 = call "scaling_calculator_baratron.vi"("x"=w539, "offset subt"="Bar_CDG1 Vbar offset") -> ("y (Pa)"=w541:dbl)  [unwired: 4 in, 1 out]
              }
              frame True {
                n223 = call "baratron_conversion_CDG1.vi"("V_CDG1 (V)"=w543) -> ("y (Pa)"=w542:dbl)  [unwired: 10 in]
              }
            }
          }
          frame #11 {
            # "11"
            # "AIN20 baratron buffer 2"
            n224 = Add Array Elements(numeric array=w544) -> (sum=w546:dbl)
            n225 = Divide(x=w546, y=w549) -> (x/y=w545:dbl)
            n226 = call "scaling_calculator_baratron.vi"("x"=w545, "offset subt"="Bar_CDG2 Vbar offset") -> ("y (Pa)"=w548:dbl)  [unwired: 4 in, 1 out]
          }
        }
        n227 = Subtract(x=w265, y=w262) -> (x-y=→"V9 - V8":dbl)
        n228 = Subtract(x=w261, y=w262) -> (x-y=→"V10 - V8":dbl)
        n229 = Subtract(x=w261, y=w264) -> (x-y=→"V10 - V9":dbl)
        n230 = Build Array(w337, w335, w333, w330, w329, w328, w326, w311, w255, w256, w257, w258) -> (w259:dbl[])
        "DAQ CONV. OUT" <- w259
        n231 = local write "OUT S.4"(w259) -> ()
        n232 = local write "OUT S.1"(w259) -> ()
        n233 = local write "OUT S.3"(w259) -> ()
        n234 = local write "OUT S.2"(w259) -> ()
        n235 = local read "current time"() -> (w309:timestamp)
        n236 = To Double Precision Float(number=w309) -> (double precision float=w352:dbl)
        n237 = Build Array (concatenate)(w339, w259) -> (w310:dbl[][])
        n238 = Index Array(array=w259) -> (element #1=w268:dbl, element #2=w278:dbl, element #3=w277:dbl, element #4=w276:dbl, element #5=w275:dbl, element #6=w274:dbl, element #7=w273:dbl, element #8=w272:dbl, element #9=w271:dbl, element #10=w270:dbl, element #11=w269:dbl, element #12=w254:dbl)  [unwired: 12 in]
        n239 = call "LV_UNIX.vi"("current time"=w309) -> ("date/time string"=w307:string, "UNIX time (s)"=w308:dbl)  [unwired: 9 in]
        n240 = local read "Cycle #"() -> (w306:i32)
        n241 = Index Array(array=w310, index (col) #1=0 ("disabled index (col)"), index (col) #2=1 ("disabled index (col)"), index (col) #3=2 ("disabled index (col)"), index (col) #4=3 ("disabled index (col)"), index (col) #5=4 ("index (col)"), index (col) #6=5 ("index (col)"), index (col) #7=6 ("index (col)"), index (col) #8=7 ("index (col)"), index (col) #9=8 ("index (col)"), index (col) #10=9 ("index (col)"), index (col) #11=10 ("index (col)"), index (col) #12=11 ("index (col)")) -> (element #1=w350:dbl[], element #2=w348:dbl[], element #3=w346:dbl[], element #4=w344:dbl[], element #5=w341:dbl[], element #6=w340:dbl[], element #7=w247:dbl[], element #8=w246:dbl[], element #9=w301:dbl[], element #10=w282:dbl[], element #11=w280:dbl[], element #12=w252:dbl[])  [unwired: 12 in]
        n242 = Bundle(w251, w350) -> (w305:cluster{dbl[], dbl[]})  [unwired: 1 in]
        n243 = Bundle(w251, w348) -> (w304:cluster{dbl[], dbl[]})  [unwired: 1 in]
        n244 = Bundle(w251, w346) -> (w300:cluster{dbl[], dbl[]})  [unwired: 1 in]
        n245 = Bundle(w251, w344) -> (w299:cluster{dbl[], dbl[]})  [unwired: 1 in]
        n246 = Bundle(w251, w341) -> (w298:cluster{dbl[], dbl[]})  [unwired: 1 in]
        n247 = Bundle(w251, w340) -> (w297:cluster{dbl[], dbl[]})  [unwired: 1 in]
        n248 = Bundle(w251, w247) -> (w296:cluster{dbl[], dbl[]})  [unwired: 1 in]
        n249 = Bundle(w251, w246) -> (w295:cluster{dbl[], dbl[]})  [unwired: 1 in]
        n250 = Bundle(w251, w301) -> (w293:cluster{dbl[], dbl[]})  [unwired: 1 in]
        n251 = Bundle(w251, w282) -> (w281:cluster{dbl[], dbl[]})  [unwired: 1 in]
        n252 = Bundle(w251, w280) -> (w279:cluster{dbl[], dbl[]})  [unwired: 1 in]
        n253 = Bundle(w251, w252) -> (w250:cluster{dbl[], dbl[]})  [unwired: 1 in]
        n254 = case shown="True" TRUE {
          tunnel: w352 -> [_ w373]
          tunnel: w308 -> [_ w374]
          tunnel: w307 -> [_ w375]
          tunnel: w306 -> [_ w376]
          tunnel: w278 -> [_ w390]
          tunnel: w277 -> [_ w389]
          tunnel: w276 -> [_ w388]
          tunnel: w275 -> [_ w387]
          tunnel: w274 -> [_ w386]
          tunnel: w273 -> [_ w385]
          tunnel: w272 -> [_ w384]
          tunnel: w271 -> [_ w383]
          tunnel: w270 -> [_ w382]
          tunnel: w269 -> [_ w381]
          tunnel: w268 -> [_ w380]
          tunnel: w254 -> [_ w359]
          frame False {
          }
          frame True {
            w379 = "%d,%s,%10.4f,%10.4f,%5.6f,%5.6f,%5.6f,%5.6f,%5.6f,%5.6f,%5.6f,%9.6f,%9.6f,%9.6f,%9.6f,%9.6f\\n" ("format string")
            n255 = local read "error out\n(file creation)"() -> (w360:errorcluster)
            n256 = local read "RAW (V)"() -> (w372:dbl[])
            n257 = local read "ref RAW"() -> (w378:refnum<file>)
            n258 = Index Array(array=w372) -> (element #1=w371:dbl, element #2=w370:dbl, element #3=w369:dbl, element #4=w368:dbl, element #5=w367:dbl, element #6=w366:dbl, element #7=w365:dbl, element #8=w364:dbl, element #9=w363:dbl, element #10=w362:dbl, element #11=w361:dbl, element #12=w358:dbl)  [unwired: 12 in]
            n259 = local read "ref DAQ"() -> (w391:refnum<file>)
            n260 = Format Into String(format string=w379, initial string=w378, error in=w360, w376, w375, w374, w373, w371, w370, w369, w368, w367, w366, w365, w364, w363, w362, w361, w358) -> (error out=w377:errorcluster)  [unwired: 1 out]
            n261 = Format Into String(format string=w379, initial string=w391, error in=w377, w376, w375, w374, w373, w380, w390, w389, w388, w387, w386, w385, w384, w383, w382, w381, w359) -> (error out=→"error out \n(record DAQ)":errorcluster)  [unwired: 1 out]
          }
        }
        n262 = Build Array(w305, w304, w300, w299, w298, w297, w296, w295, w293, w281, w279, w250) -> (w292:cluster{dbl[], dbl[]}[])
        n263 = stacked-sequence {
          tunnel: w292 -> [w397 w409 w421 w433]
          frame #0 {
            n264 = local read "NI-DAQ CH indic."() -> (w394:string[])
            n265 = control-ref of="XY Graph S.1"() -> (w395:refnum<vi>)
            n266 = Array Size(array=w394) -> (size(s)=w396:i32)
            n267 = for {
              N: w396 -> [_]
              tunnel: w395 -> [w403]
              tunnel: w394 -> [w401] mode=indexing
              tunnel: [w400] -> w393
              i -> [w404]
              n268 = property class="XYGraph (strict)"(reference=w403, error in=errorcluster {"status"=FALSE, "code"=0, "source"=""} ("error in (no error)"), "Active Plot"=w404, "Plot.Plot Name"=w401) -> (error out=w400:errorcluster)  [unwired: 1 out]
            }
            n269 = property class="XYGraph (strict)"(reference=w395, error in=w393, "Val(Sgnl)"=w397) -> (error out=w398:errorcluster)  [unwired: 1 out]
            n270 = control-ref of="error plot content"() -> (w399:refnum<vi>)
            n271 = property class="Clust (strict)"(reference=w399, "Value"=w398) -> ()  [unwired: 1 in, 2 out]
          }
          frame #1 {
            n272 = local read "NI-DAQ CH indic."() -> (w407:string[])
            n273 = control-ref of="XY Graph S.2"() -> (w405:refnum<vi>)
            n274 = Array Size(array=w407) -> (size(s)=w408:i32)
            n275 = for {
              N: w408 -> [_]
              tunnel: w405 -> [w415]
              tunnel: w407 -> [w413] mode=indexing
              tunnel: [w412] -> w406
              i -> [w416]
              n276 = property class="XYGraph (strict)"(reference=w415, error in=errorcluster {"status"=FALSE, "code"=0, "source"=""} ("error in (no error)"), "Active Plot"=w416, "Plot.Plot Name"=w413) -> (error out=w412:errorcluster)  [unwired: 1 out]
            }
            n277 = property class="XYGraph (strict)"(reference=w405, error in=w406, "Val(Sgnl)"=w409) -> (error out=w410:errorcluster)  [unwired: 1 out]
            n278 = control-ref of="error plot content"() -> (w411:refnum<vi>)
            n279 = property class="Clust (strict)"(reference=w411, "Value"=w410) -> ()  [unwired: 1 in, 2 out]
          }
          frame #2 {
            n280 = local read "NI-DAQ CH indic."() -> (w419:string[])
            n281 = control-ref of="XY Graph S.3"() -> (w417:refnum<vi>)
            n282 = Array Size(array=w419) -> (size(s)=w420:i32)
            n283 = for {
              N: w420 -> [_]
              tunnel: w417 -> [w427]
              tunnel: w419 -> [w425] mode=indexing
              tunnel: [w424] -> w418
              i -> [w428]
              n284 = property class="XYGraph (strict)"(reference=w427, error in=errorcluster {"status"=FALSE, "code"=0, "source"=""} ("error in (no error)"), "Active Plot"=w428, "Plot.Plot Name"=w425) -> (error out=w424:errorcluster)  [unwired: 1 out]
            }
            n285 = property class="XYGraph (strict)"(reference=w417, error in=w418, "Val(Sgnl)"=w421) -> (error out=w422:errorcluster)  [unwired: 1 out]
            n286 = control-ref of="error plot content"() -> (w423:refnum<vi>)
            n287 = property class="Clust (strict)"(reference=w423, "Value"=w422) -> ()  [unwired: 1 in, 2 out]
          }
          frame #3 {
            n288 = local read "NI-DAQ CH indic."() -> (w431:string[])
            n289 = control-ref of="XY Graph S.4"() -> (w429:refnum<vi>)
            n290 = Array Size(array=w431) -> (size(s)=w432:i32)
            n291 = for {
              N: w432 -> [_]
              tunnel: w429 -> [w439]
              tunnel: w431 -> [w437] mode=indexing
              tunnel: [w436] -> w430
              i -> [w440]
              n292 = property class="XYGraph (strict)"(reference=w439, error in=errorcluster {"status"=FALSE, "code"=0, "source"=""} ("error in (no error)"), "Active Plot"=w440, "Plot.Plot Name"=w437) -> (error out=w436:errorcluster)  [unwired: 1 out]
            }
            n293 = property class="XYGraph (strict)"(reference=w429, error in=w430, "Val(Sgnl)"=w433) -> (error out=w434:errorcluster)  [unwired: 1 out]
            n294 = control-ref of="error plot content"() -> (w435:refnum<vi>)
            n295 = property class="Clust (strict)"(reference=w435, "Value"=w434) -> ()  [unwired: 1 in, 2 out]
          }
        }
      }
      frame #1 {
        n296 = local read "error out \n(DAQ IN)"() -> (w551:errorcluster)
        n297 = local read "DAQ OUT ON?"() -> (w553:bool)
        n298 = case shown="True" w553 {
          tunnel: w554 -> [w556 w561]
          tunnel: [w556 w560] -> w552
          tunnel: w551 -> [w555 w558]
          tunnel: [w555 w557] -> w550
          frame False {
          }
          frame True {
            n299 = call <vilib>:"DAQmx Write (Analog 1D DBL 1Chan NSamp).vi"("task/channels in"=w561, "data"="DAQ OUT SET Volt", "timeout"=100.0, "error in"=w558) -> ("task out"=w560:refnum<k21>, "number of samples written per channel"=→"DAQ OUT \nsample #":u32, "error out"=w557:errorcluster)  [unwired: 9 in]
          }
        }
        "error out\n(DAQ OUT)" <- w550
      }
    }
    "Cycle #" <- w240
  }
  n300 = call <vilib>:"DAQmx Stop Task.vi"("task/channels in"=w12, "error in"=w10) -> ("task out"=w14:refnum<k21>, "error out"=w13:errorcluster)  [unwired: 12 in]
  n301 = call <vilib>:"DAQmx Clear Task.vi"("task in"=w14, "error in"=w13) -> ("error out"=w16:errorcluster)  [unwired: 13 in]
  n302 = call <vilib>:"DAQmx Stop Task.vi"("task/channels in"=w11, "error in"=w16) -> ("task out"=w18:refnum<k21>, "error out"=w15:errorcluster)  [unwired: 12 in]
  n303 = call <vilib>:"DAQmx Clear Task.vi"("task in"=w18, "error in"=w15) -> ("error out"=→"error out DAQ close":errorcluster)  [unwired: 13 in]
